vi "Main.vi"() -> ()   [LabVIEW 2013]
uses:
  <vilib>/Utility/miscctls.llb/LVFontTypeDef.ctl
panel:
  out "текущий ист.":u8
  in  "SetCurrent":dbl min=0.0 max=72.0 step=0.1 format="%#.1g"
  in  "SetVoltage":dbl min=0.0 max=30.0 step=0.1 format="%#.1g"
  in  "SetCurrentB":bool
  in  "SetVoltageB":bool
  in  "SetOutputOffB":bool
  in  "SetOutputOnB":bool
  in  "ConnectChannel":bool
  in  "DisconnectChannel":bool
  in  "Comm. current %":dbl=0.5 caption="%" min=0.0 max=100.0 step=0.5
  in  "Common curr. dec":bool
  in  "Common curr. inc":bool
  in  "ConnectAll":bool
  in  "DisconnectAll":bool
  in  "Set Output ON All":bool caption="ВЫХОДЫ ИСТОЧНИКОВ"
  in  "SetCurrentAll":bool
  in  "SetVoltageAll":bool
  out "Дата":string
  out "Время":string
  in  "Comm. voltage %":dbl caption="%" min=0.0 max=100.0 step=0.5
  in  "Common volt. dec":bool
  in  "Common volt. inc":bool
  in  "ReadFromFile":bool
  in  "WriteToFile":bool
  in  "№":string="55"
  in  "DeleteChannel":bool
  in  "IP":string="172.16.21.19"
  in  "AddChannel":bool
  out "CURRENTSET":dbl[](array[numeric])
  in  "CurrentModulationOn":bool
  in  "Amp":dbl
  in  "CurrentModulationB":bool
  out "NAME":string[](array[string])
  out "ADRESS":string[](array[string])
  out "VIRef":refnum<vi>[](array[refnum])
  in  "Quit":bool
  in  "List of channels":i32(listbox)
  # "ИСТОЧНИК №_"
  # "ВСЕ ИСТОЧНИКИ"
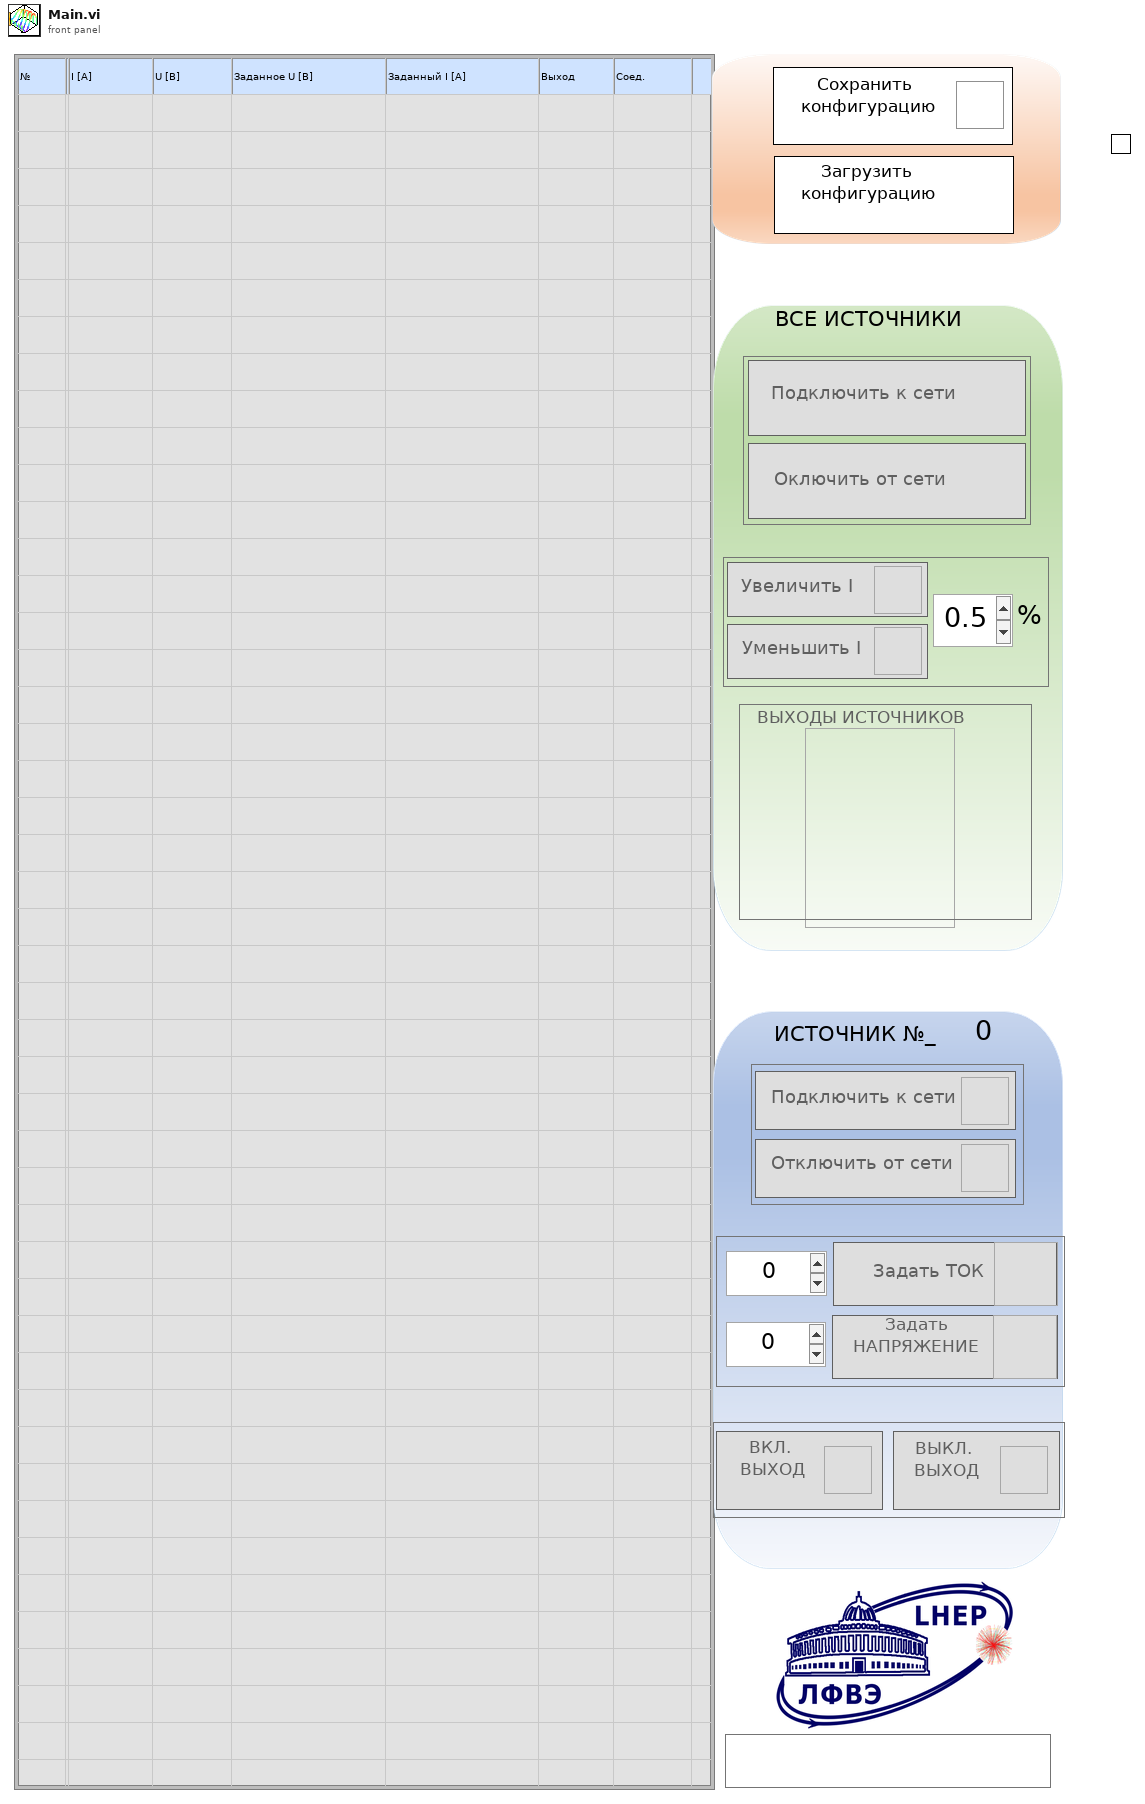
[diagram p1: front panel]
types:
  T1 = enum8{"Enabled", "Disabled", "Disabled and Grayed Out"}
  T2 = typedef "LVFontTypeDef.ctl" = cluster{"Font Name":string, "Size":u16, "Bold":bool, "Italic":bool, "Underline":bool, "Strikeout":bool, "Color":u32}
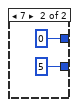
[diagram p4: hidden frame]
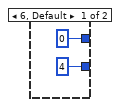
[diagram p5: hidden frame]
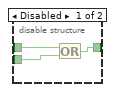
[diagram p6: hidden frame]
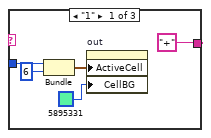
[diagram p7: hidden frame]
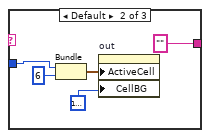
[diagram p8: hidden frame]
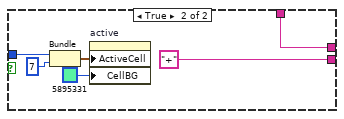
[diagram p9: hidden frame]
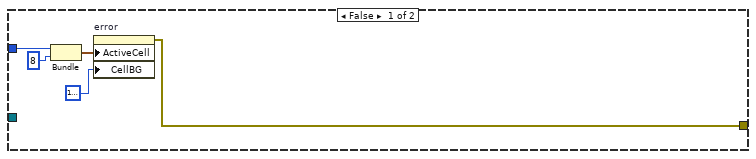
[diagram p10: hidden frame]
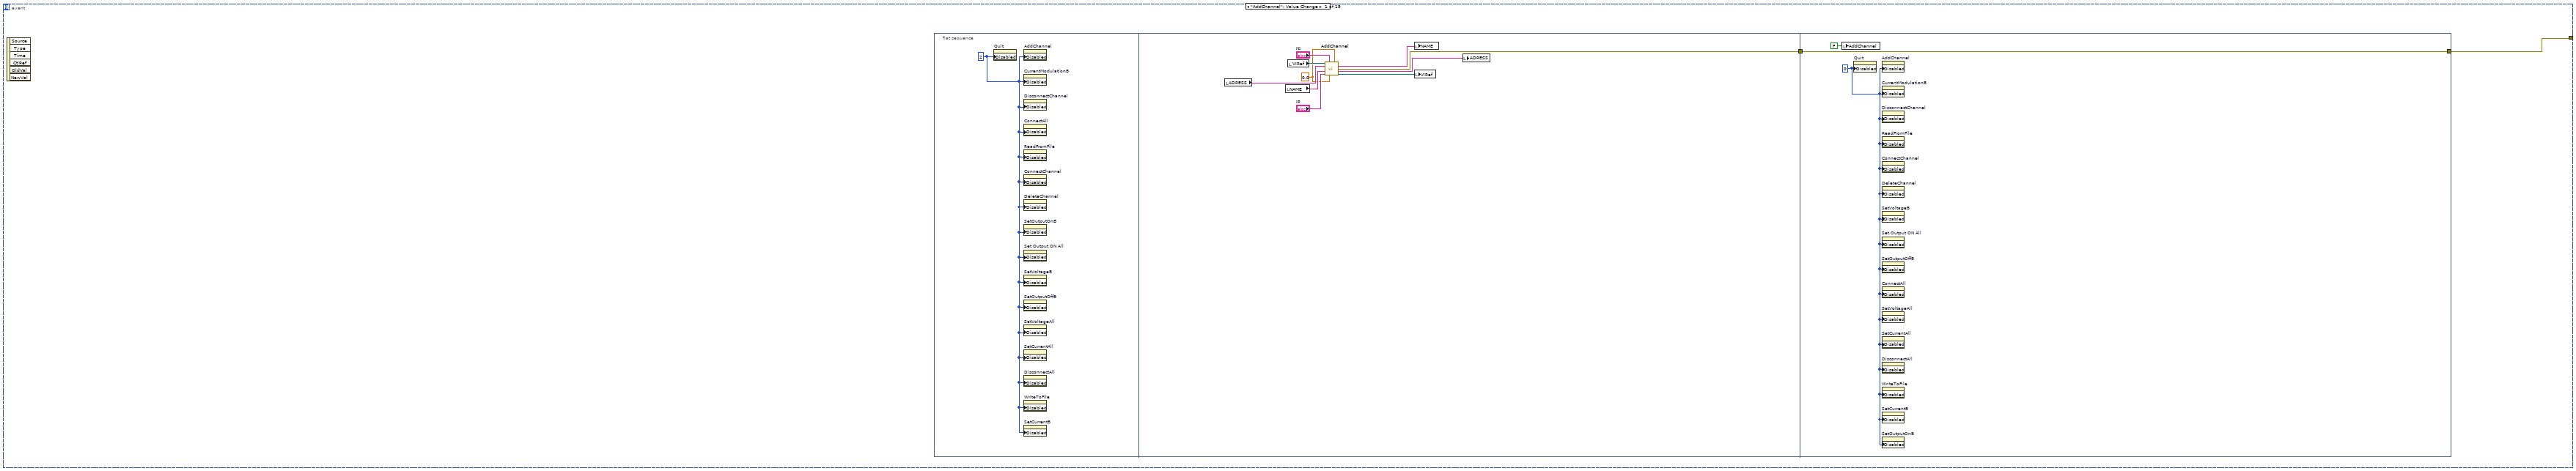
[diagram p11: hidden frame]
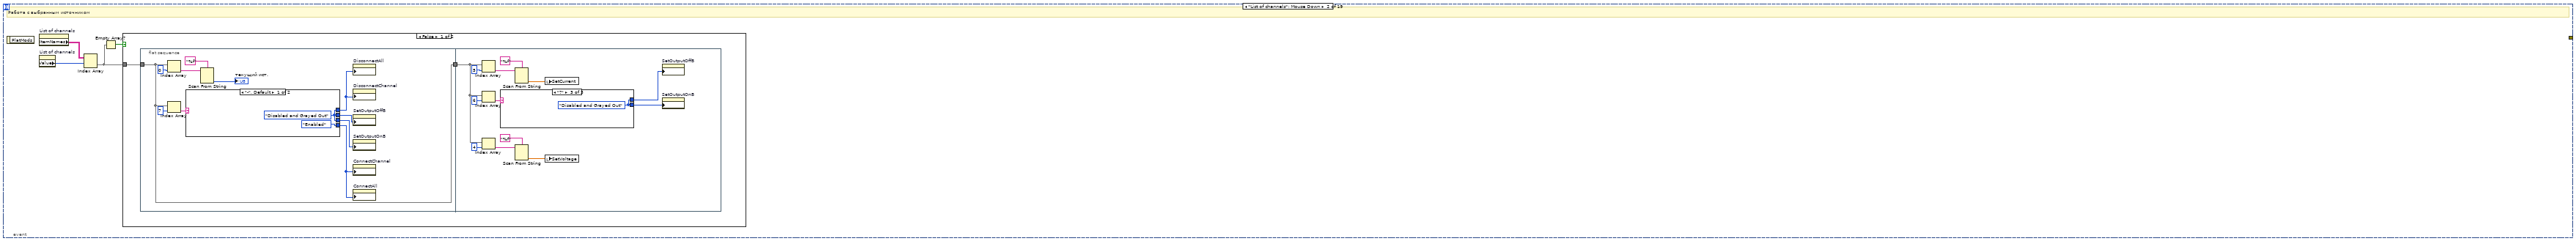
[diagram p12: hidden frame]
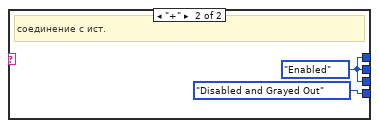
[diagram p13: hidden frame]
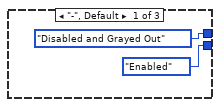
[diagram p14: hidden frame]
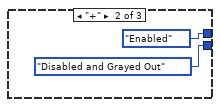
[diagram p15: hidden frame]
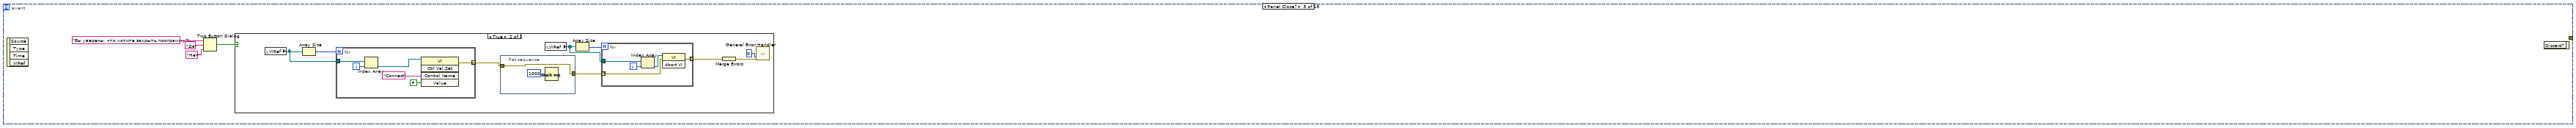
[diagram p17: hidden frame]
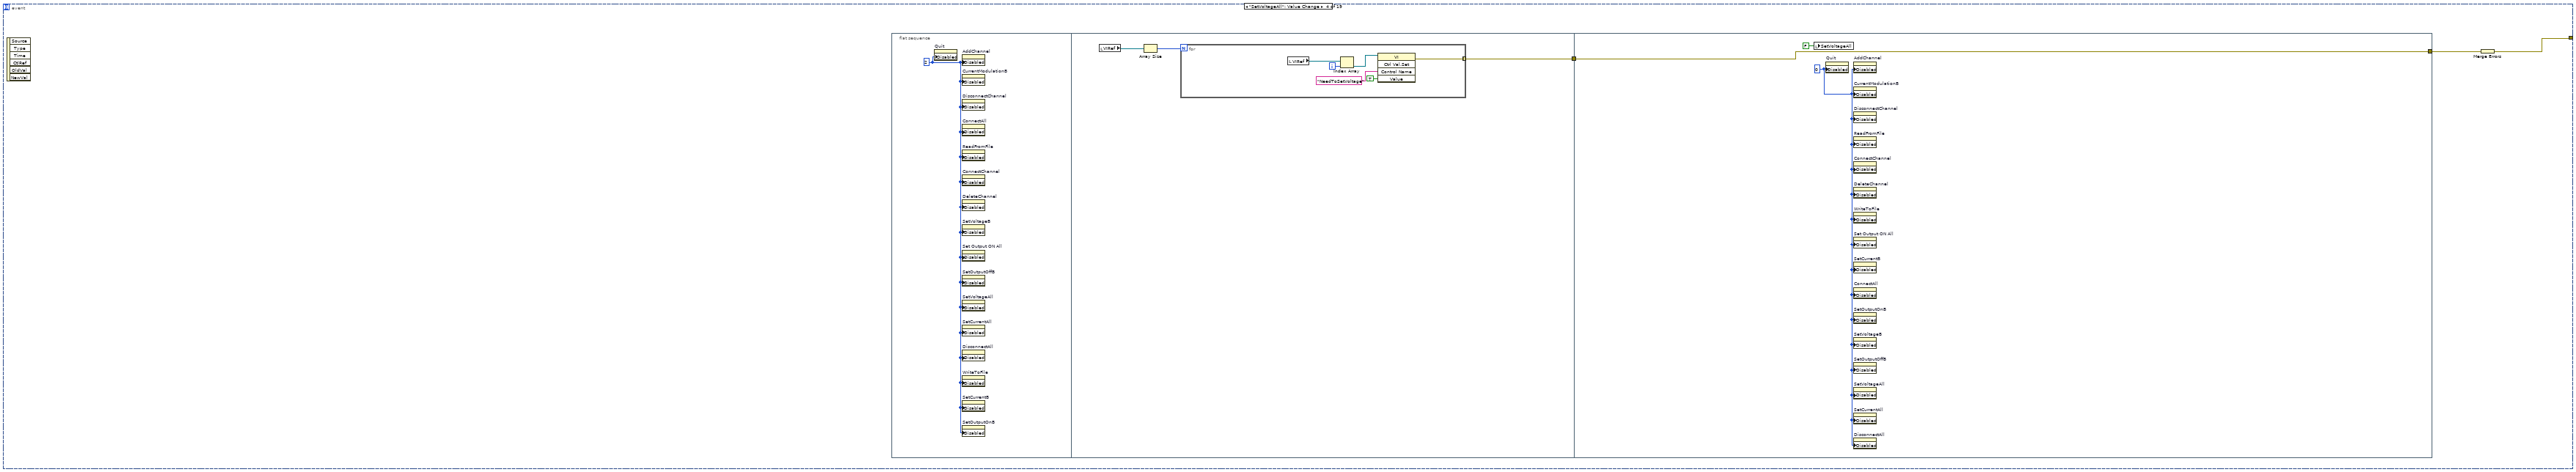
[diagram p19: hidden frame]
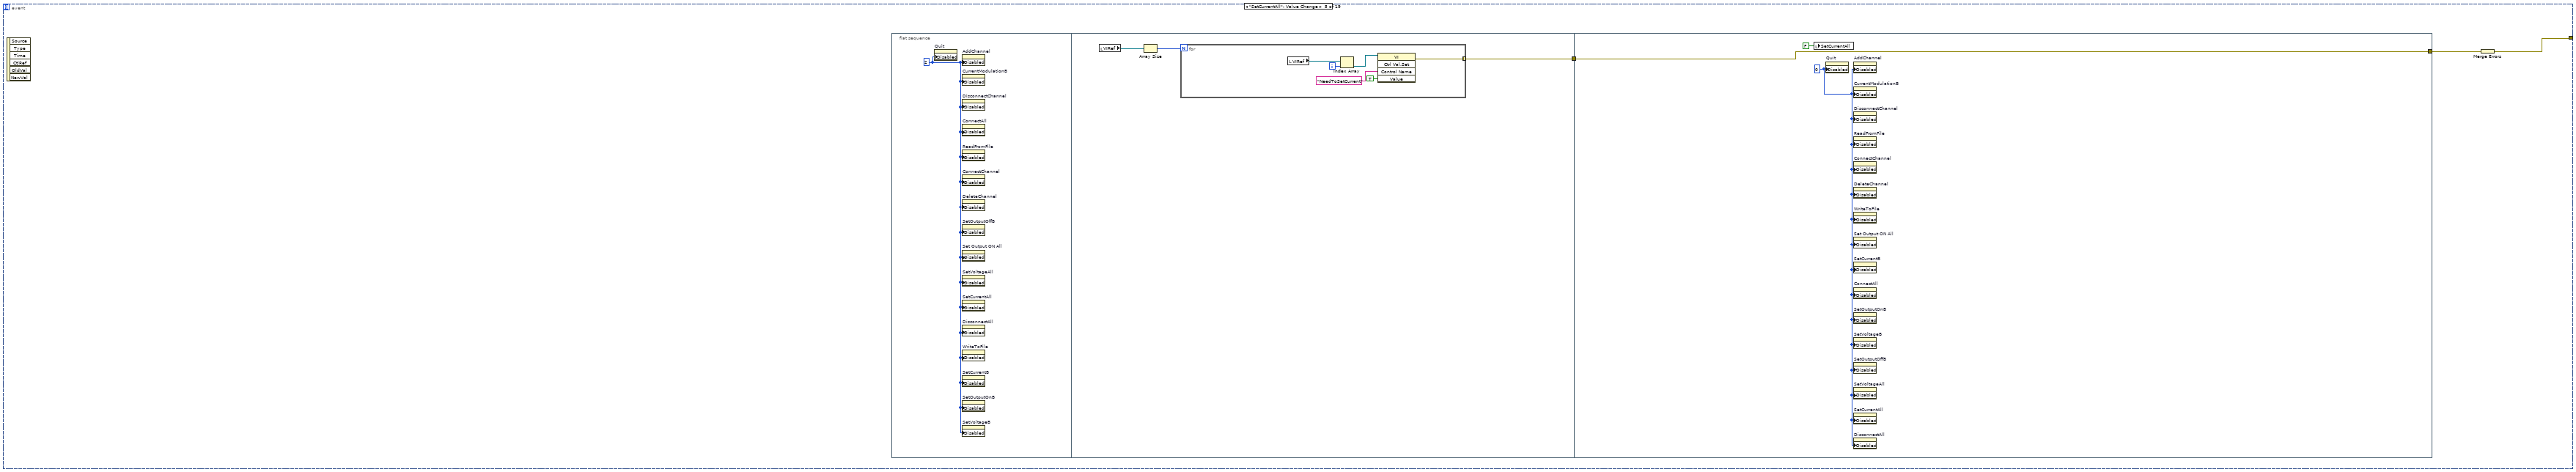
[diagram p20: hidden frame]
diagram:
  w19 = u8 0 ("Disabled")
  w21 = FALSE ("SetOutputOnB")
  w22 = FALSE ("OK Button")
  n1 = event shown="[0] \"Quit\": Value Change" {
    selector: _ -> [_]
    dyn-events: _ -> [_]
    timeout: _ -> [_]
    event "Quit": Value Change {
      n2 = event-data() -> ()  [unwired: 1 in, 5 out]
      n3 = Stop(stop? (T)=TRUE) -> ()
    }
  }
  n4 = while {
    stop <- FALSE stop-if-true
    n5 = property on="List of channels" class="MCListbox (strict)"() -> ("ItemNames"=w33:string[][])  [unwired: 2 in, 2 out]
    n6 = Get Date/Time String(want seconds? (F)=TRUE) -> (date string=→"Дата":string, time string=→"Время":string)  [unwired: 2 in]
    n7 = Wait Until Next ms Multiple(millisecond multiple=u16 1000) -> ()  [unwired: 1 out]
    n8 = Empty Array?(array=w33) -> (empty?=w32:bool)
    n9 = case shown="True" w32 {
      frame False {
      }
      frame True {
        w35 = T1."Disabled and Grayed Out" ("Disabled")
        n10 = property on="Common curr. inc" class="Bool (strict)"("DisabledEnum"=w35) -> ()  [unwired: 2 in, 2 out]
        n11 = property on="Common curr. dec" class="Bool (strict)"("DisabledEnum"=w35) -> ()  [unwired: 2 in, 2 out]
        n12 = property on="Set Output ON All" class="Bool (strict)"("DisabledEnum"=w35) -> ()  [unwired: 2 in, 2 out]
        n13 = property on="Common volt. inc" class="Bool (strict)"("DisabledEnum"=w35) -> ()  [unwired: 2 in, 2 out]
        n14 = property on="DisconnectAll" class="Bool (strict)"("DisabledEnum"=w35) -> ()  [unwired: 2 in, 2 out]
        n15 = property on="SetVoltageB" class="Bool (strict)"("DisabledEnum"=w35) -> ()  [unwired: 2 in, 2 out]
        n16 = property on="ConnectChannel" class="Bool (strict)"("DisabledEnum"=w35) -> ()  [unwired: 2 in, 2 out]
        n17 = property on="SetOutputOnB" class="Bool (strict)"("DisabledEnum"=w35) -> ()  [unwired: 2 in, 2 out]
        n18 = property on="DisconnectChannel" class="Bool (strict)"("DisabledEnum"=w35) -> ()  [unwired: 2 in, 2 out]
        n19 = property on="SetOutputOffB" class="Bool (strict)"("DisabledEnum"=w35) -> ()  [unwired: 2 in, 2 out]
        n20 = property on="ConnectAll" class="Bool (strict)"("DisabledEnum"=w35) -> ()  [unwired: 2 in, 2 out]
        n21 = property on="SetCurrentB" class="Bool (strict)"("DisabledEnum"=w35) -> ()  [unwired: 2 in, 2 out]
      }
    }
  }
  n22 = while {
    stop <- FALSE stop-if-true
    n23 = event shown="[15] \"WriteToFile\": Value Change" {
      selector: _ -> [_ _ _ _ _ _ _ _ _ _ _ _ _ _ _ _ _ _ _]
      dyn-events: _ -> [_ _ _ _ _ _ _ _ _ _ _ _ _ _ _ _ _ _ _]
      timeout: _ -> [_ _ _ _ _ _ _ _ _ _ _ _ _ _ _ _ _ _ _]
      tunnel: [w39 _ _ w120 w136 w152 w196 w240 w255 w281 w297 w313 w330 w351 w374 w392 w443 w517 w540] -> w36
      event "AddChannel": Value Change {
        n24 = event-data() -> ()  [unwired: 7 out]
        n25 = flat-sequence {
          tunnel: [w42] -> w40
          tunnel: [w52] -> w39
          tunnel: w40 -> [w52]
          frame #0 {
            w41 = u8 2 ("Disabled")
            n26 = property on="Quit" class="Bool (strict)"("Disabled"=w41) -> ()  [unwired: 2 in, 2 out]
            n27 = property on="AddChannel" class="Bool (strict)"("Disabled"=w41) -> ()  [unwired: 2 in, 2 out]
            n28 = property on="CurrentModulationB" class="Bool (strict)"("Disabled"=w41) -> ()  [unwired: 2 in, 2 out]
            n29 = property on="DisconnectChannel" class="Bool (strict)"("Disabled"=w41) -> ()  [unwired: 2 in, 2 out]
            n30 = property on="ConnectAll" class="Bool (strict)"("Disabled"=w41) -> ()  [unwired: 2 in, 2 out]
            n31 = property on="ReadFromFile" class="Bool (strict)"("Disabled"=w41) -> ()  [unwired: 2 in, 2 out]
            n32 = property on="ConnectChannel" class="Bool (strict)"("Disabled"=w41) -> ()  [unwired: 2 in, 2 out]
            n33 = property on="DeleteChannel" class="Bool (strict)"("Disabled"=w41) -> ()  [unwired: 2 in, 2 out]
            n34 = property on="SetOutputOnB" class="Bool (strict)"("Disabled"=w41) -> ()  [unwired: 2 in, 2 out]
            n35 = property on="Set Output ON All" class="Bool (strict)"("Disabled"=w41) -> ()  [unwired: 2 in, 2 out]
            n36 = property on="SetVoltageB" class="Bool (strict)"("Disabled"=w41) -> ()  [unwired: 2 in, 2 out]
            n37 = property on="SetOutputOffB" class="Bool (strict)"("Disabled"=w41) -> ()  [unwired: 2 in, 2 out]
            n38 = property on="SetVoltageAll" class="Bool (strict)"("Disabled"=w41) -> ()  [unwired: 2 in, 2 out]
            n39 = property on="SetCurrentAll" class="Bool (strict)"("Disabled"=w41) -> ()  [unwired: 2 in, 2 out]
            n40 = property on="DisconnectAll" class="Bool (strict)"("Disabled"=w41) -> ()  [unwired: 2 in, 2 out]
            n41 = property on="WriteToFile" class="Bool (strict)"("Disabled"=w41) -> ()  [unwired: 2 in, 2 out]
            n42 = property on="SetCurrentB" class="Bool (strict)"("Disabled"=w41) -> ()  [unwired: 2 in, 2 out]
          }
          frame #1 {
            w43 = 0.0 ("SetVoltage")
            n43 = local read "ADRESS"() -> (w49:string[])
            n44 = local read "NAME"() -> (w48:string[])
            n45 = local read "VIRef"() -> (w47:refnum<vi>[])
            n46 = call "AddChannel.vi"("VIRef"=w47, "Name"="№", "SetCurrent"=w43, "ADRESS"=w49, "NAME"=w48, "Address"="IP", "SetVoltage"=w43) -> ("NAMEOut"=w44:string[], "error out"=w42:errorcluster, "ADRESSOut"=w45:string[], "VIRefOut"=w46:refnum<vi>[])  [unwired: 1 in, 4 out]
            n47 = local write "NAME"(w44) -> ()
            n48 = local write "VIRef"(w46) -> ()
            n49 = local write "ADRESS"(w45) -> ()
          }
          frame #2 {
            w53 = u8 0 ("Disabled")
            n50 = local write "AddChannel"(FALSE ("AddChannel")) -> ()
            n51 = property on="Quit" class="Bool (strict)"("Disabled"=w53) -> ()  [unwired: 2 in, 2 out]
            n52 = property on="AddChannel" class="Bool (strict)"("Disabled"=w53) -> ()  [unwired: 2 in, 2 out]
            n53 = property on="CurrentModulationB" class="Bool (strict)"("Disabled"=w53) -> ()  [unwired: 2 in, 2 out]
            n54 = property on="DisconnectChannel" class="Bool (strict)"("Disabled"=w53) -> ()  [unwired: 2 in, 2 out]
            n55 = property on="ReadFromFile" class="Bool (strict)"("Disabled"=w53) -> ()  [unwired: 2 in, 2 out]
            n56 = property on="ConnectChannel" class="Bool (strict)"("Disabled"=w53) -> ()  [unwired: 2 in, 2 out]
            n57 = property on="DeleteChannel" class="Bool (strict)"("Disabled"=w53) -> ()  [unwired: 2 in, 2 out]
            n58 = property on="SetVoltageB" class="Bool (strict)"("Disabled"=w53) -> ()  [unwired: 2 in, 2 out]
            n59 = property on="Set Output ON All" class="Bool (strict)"("Disabled"=w53) -> ()  [unwired: 2 in, 2 out]
            n60 = property on="SetOutputOffB" class="Bool (strict)"("Disabled"=w53) -> ()  [unwired: 2 in, 2 out]
            n61 = property on="ConnectAll" class="Bool (strict)"("Disabled"=w53) -> ()  [unwired: 2 in, 2 out]
            n62 = property on="SetVoltageAll" class="Bool (strict)"("Disabled"=w53) -> ()  [unwired: 2 in, 2 out]
            n63 = property on="SetCurrentAll" class="Bool (strict)"("Disabled"=w53) -> ()  [unwired: 2 in, 2 out]
            n64 = property on="DisconnectAll" class="Bool (strict)"("Disabled"=w53) -> ()  [unwired: 2 in, 2 out]
            n65 = property on="WriteToFile" class="Bool (strict)"("Disabled"=w53) -> ()  [unwired: 2 in, 2 out]
            n66 = property on="SetCurrentB" class="Bool (strict)"("Disabled"=w53) -> ()  [unwired: 2 in, 2 out]
            n67 = property on="SetOutputOnB" class="Bool (strict)"("Disabled"=w53) -> ()  [unwired: 2 in, 2 out]
          }
        }
      }
      event "List of channels": Mouse Down {
        # "Работа с выбранным источником"
        n68 = event-data() -> ()  [unwired: 2 out]
        n69 = property on="List of channels" class="MCListbox (strict)"() -> ("ItemNames"=w58:string[][])  [unwired: 2 in, 2 out]
        n70 = property on="List of channels" class="MCListbox (strict)"() -> ("Value"=w57:i32)  [unwired: 2 in, 2 out]
        n71 = Index Array(array=w58, index (row)=w57) -> (element=w56:string[])  [unwired: 1 in]
        n72 = Empty Array?(array=w56) -> (empty?=w55:bool)
        n73 = case shown="False" w55 {
          tunnel: w56 -> [w59 _]
          frame False {
            n74 = flat-sequence {
              tunnel: w59 -> [w65]
              tunnel: [w65] -> w60
              tunnel: w60 -> [w76]
              frame #0 {
                n75 = Index Array(array=w65, index=0) -> (element=w68:string)
                n76 = Index Array(array=w65, index=7) -> (element=w66:string)
                n77 = case shown="\"-\", Default" w66 {
                  tunnel: [T1."Enabled" ("Disabled") T1."Disabled and Grayed Out" ("Disabled")] -> w61
                  tunnel: [w72 w74] -> w62
                  tunnel: [w72 w74] -> w64
                  tunnel: [w72 w74] -> w63
                  frame "-", Default {
                    w72 = T1."Disabled and Grayed Out" ("Disabled")
                  }
                  frame "+" {
                    w74 = T1."Enabled" ("Disabled")
                    # "соединение с ист."
                  }
                }
                n78 = Scan From String(format string="%f", input string=w68) -> (output 1=→"текущий ист.":u8)  [unwired: 3 in, 3 out]
                n79 = property on="DisconnectAll" class="Bool (strict)"("DisabledEnum"=w62) -> ()  [unwired: 2 in, 2 out]
                n80 = property on="DisconnectChannel" class="Bool (strict)"("DisabledEnum"=w62) -> ()  [unwired: 2 in, 2 out]
                n81 = property on="SetOutputOffB" class="Bool (strict)"("DisabledEnum"=w64) -> ()  [unwired: 2 in, 2 out]
                n82 = property on="SetOutputOnB" class="Bool (strict)"("DisabledEnum"=w63) -> ()  [unwired: 2 in, 2 out]
                n83 = property on="ConnectChannel" class="Bool (strict)"("DisabledEnum"=w61) -> ()  [unwired: 2 in, 2 out]
                n84 = property on="ConnectAll" class="Bool (strict)"("DisabledEnum"=w61) -> ()  [unwired: 2 in, 2 out]
              }
              frame #1 {
                n85 = Index Array(array=w76, index=5) -> (element=w82:string)
                n86 = Index Array(array=w76, index=6) -> (element=w86:string)
                n87 = Index Array(array=w76, index=4) -> (element=w78:string)
                n88 = case shown="\"?\"" w86 {
                  tunnel: [T1."Enabled" ("Disabled") T1."Disabled and Grayed Out" ("Disabled") w93] -> w87
                  tunnel: [T1."Disabled and Grayed Out" ("Disabled") T1."Enabled" ("Disabled") w93] -> w88
                  frame "-", Default {
                  }
                  frame "+" {
                  }
                  frame "?" {
                    w93 = T1."Disabled and Grayed Out" ("Disabled")
                  }
                }
                n89 = Scan From String(format string="%f", input string=w82) -> (output 1=w84:dbl)  [unwired: 3 in, 3 out]
                n90 = Scan From String(format string="%f", input string=w78) -> (output 1=w79:dbl)  [unwired: 3 in, 3 out]
                n91 = local write "SetCurrent"(w84) -> ()
                n92 = local write "SetVoltage"(w79) -> ()
                n93 = property on="SetOutputOffB" class="Bool (strict)"("DisabledEnum"=w88) -> ()  [unwired: 2 in, 2 out]
                n94 = property on="SetOutputOnB" class="Bool (strict)"("DisabledEnum"=w87) -> ()  [unwired: 2 in, 2 out]
              }
            }
          }
          frame True {
          }
        }
      }
      event Panel Close? {
        n95 = event-data() -> ()  [unwired: 5 out]
        n96 = Two Button Dialog(message="Вы уверены, что хотите закрыть программу?", 1:"Нет" ("F button name (\"Cancel\")"), 2:"Да" ("T button name (\"OK\")")) -> (T button?=w97:bool)
        n97 = case shown="True" w97 {
          frame False {
          }
          frame True {
            n98 = local read "VIRef"() -> (w99:refnum<vi>[])
            n99 = Array Size(array=w99) -> (size(s)=w98:i32)
            n100 = for {
              N: w98 -> [_]
              tunnel: w99 -> [w116]
              tunnel: [w114] -> w106 mode=indexing
              i -> [w117]
              n101 = Index Array(array=w116, index=w117) -> (element=w115:refnum<vi>)
              n102 = invoke class="VI" method="Ctrl Val.Set"(reference=w115, "Control Name"="Connect", "Value"=FALSE) -> (error out=w114:errorcluster)  [unwired: 2 in, 4 out]
            }
            n103 = flat-sequence {
              tunnel: [w108] -> w105
              tunnel: w106 -> [w108]
              frame #0 {
                n104 = Wait (ms)(milliseconds to wait=u32 1000) -> ()  [unwired: 1 out]
              }
            }
            n105 = local read "VIRef"() -> (w100:refnum<vi>[])
            n106 = Array Size(array=w100) -> (size(s)=w101:i32)
            n107 = for {
              N: w101 -> [_]
              tunnel: w100 -> [w112]
              tunnel: [w110] -> w102 mode=indexing
              tunnel: w105 -> [w109] mode=indexing
              i -> [w113]
              n108 = Index Array(array=w112, index=w113) -> (element=w111:refnum<vi>)
              n109 = invoke class="VI" method="Abort VI"(reference=w111, error in=w109) -> (error out=w110:errorcluster)  [unwired: 1 in, 2 out]
            }
            n110 = Merge Errors(w102) -> (w103:errorcluster)
            n111 = call <vilib>:"General Error Handler.vi"("type of dialog (OK msg:1)"=u32 0 ("milliseconds to wait"), "error in (no error)"=w103) -> ()  [unwired: 9 in, 5 out]
          }
        }
        n112 = event-data() -> ()  [unwired: 2 in, 1 out]
      }
      event "SetVoltageAll": Value Change {
        n113 = event-data() -> ()  [unwired: 7 out]
        n114 = flat-sequence {
          tunnel: [w124] -> w122
          tunnel: [w133] -> w121
          tunnel: w122 -> [w133]
          frame #0 {
            w123 = u8 2 ("Disabled")
            n115 = property on="Quit" class="Bool (strict)"("Disabled"=w123) -> ()  [unwired: 2 in, 2 out]
            n116 = property on="AddChannel" class="Bool (strict)"("Disabled"=w123) -> ()  [unwired: 2 in, 2 out]
            n117 = property on="CurrentModulationB" class="Bool (strict)"("Disabled"=w123) -> ()  [unwired: 2 in, 2 out]
            n118 = property on="DisconnectChannel" class="Bool (strict)"("Disabled"=w123) -> ()  [unwired: 2 in, 2 out]
            n119 = property on="ConnectAll" class="Bool (strict)"("Disabled"=w123) -> ()  [unwired: 2 in, 2 out]
            n120 = property on="ReadFromFile" class="Bool (strict)"("Disabled"=w123) -> ()  [unwired: 2 in, 2 out]
            n121 = property on="ConnectChannel" class="Bool (strict)"("Disabled"=w123) -> ()  [unwired: 2 in, 2 out]
            n122 = property on="DeleteChannel" class="Bool (strict)"("Disabled"=w123) -> ()  [unwired: 2 in, 2 out]
            n123 = property on="SetVoltageB" class="Bool (strict)"("Disabled"=w123) -> ()  [unwired: 2 in, 2 out]
            n124 = property on="Set Output ON All" class="Bool (strict)"("Disabled"=w123) -> ()  [unwired: 2 in, 2 out]
            n125 = property on="SetOutputOffB" class="Bool (strict)"("Disabled"=w123) -> ()  [unwired: 2 in, 2 out]
            n126 = property on="SetVoltageAll" class="Bool (strict)"("Disabled"=w123) -> ()  [unwired: 2 in, 2 out]
            n127 = property on="SetCurrentAll" class="Bool (strict)"("Disabled"=w123) -> ()  [unwired: 2 in, 2 out]
            n128 = property on="DisconnectAll" class="Bool (strict)"("Disabled"=w123) -> ()  [unwired: 2 in, 2 out]
            n129 = property on="WriteToFile" class="Bool (strict)"("Disabled"=w123) -> ()  [unwired: 2 in, 2 out]
            n130 = property on="SetCurrentB" class="Bool (strict)"("Disabled"=w123) -> ()  [unwired: 2 in, 2 out]
            n131 = property on="SetOutputOnB" class="Bool (strict)"("Disabled"=w123) -> ()  [unwired: 2 in, 2 out]
          }
          frame #1 {
            n132 = local read "VIRef"() -> (w126:refnum<vi>[])
            n133 = Array Size(array=w126) -> (size(s)=w125:i32)
            n134 = for {
              N: w125 -> [_]
              tunnel: [w127] -> w124 mode=indexing
              i -> [w129]
              n135 = local read "VIRef"() -> (w132:refnum<vi>[])
              n136 = Index Array(array=w132, index=w129) -> (element=w128:refnum<vi>)
              n137 = invoke class="VI" method="Ctrl Val.Set"(reference=w128, "Control Name"="NeedToSetVoltage", "Value"=TRUE ("ConnectChannel")) -> (error out=w127:errorcluster)  [unwired: 2 in, 4 out]
            }
          }
          frame #2 {
            w134 = u8 0 ("Disabled")
            n138 = local write "SetVoltageAll"(FALSE ("SetVoltageAll")) -> ()
            n139 = property on="Quit" class="Bool (strict)"("Disabled"=w134) -> ()  [unwired: 2 in, 2 out]
            n140 = property on="AddChannel" class="Bool (strict)"("Disabled"=w134) -> ()  [unwired: 2 in, 2 out]
            n141 = property on="CurrentModulationB" class="Bool (strict)"("Disabled"=w134) -> ()  [unwired: 2 in, 2 out]
            n142 = property on="DisconnectChannel" class="Bool (strict)"("Disabled"=w134) -> ()  [unwired: 2 in, 2 out]
            n143 = property on="ReadFromFile" class="Bool (strict)"("Disabled"=w134) -> ()  [unwired: 2 in, 2 out]
            n144 = property on="ConnectChannel" class="Bool (strict)"("Disabled"=w134) -> ()  [unwired: 2 in, 2 out]
            n145 = property on="DeleteChannel" class="Bool (strict)"("Disabled"=w134) -> ()  [unwired: 2 in, 2 out]
            n146 = property on="WriteToFile" class="Bool (strict)"("Disabled"=w134) -> ()  [unwired: 2 in, 2 out]
            n147 = property on="Set Output ON All" class="Bool (strict)"("Disabled"=w134) -> ()  [unwired: 2 in, 2 out]
            n148 = property on="SetCurrentB" class="Bool (strict)"("Disabled"=w134) -> ()  [unwired: 2 in, 2 out]
            n149 = property on="ConnectAll" class="Bool (strict)"("Disabled"=w134) -> ()  [unwired: 2 in, 2 out]
            n150 = property on="SetOutputOnB" class="Bool (strict)"("Disabled"=w134) -> ()  [unwired: 2 in, 2 out]
            n151 = property on="SetVoltageB" class="Bool (strict)"("Disabled"=w134) -> ()  [unwired: 2 in, 2 out]
            n152 = property on="SetOutputOffB" class="Bool (strict)"("Disabled"=w134) -> ()  [unwired: 2 in, 2 out]
            n153 = property on="SetVoltageAll" class="Bool (strict)"("Disabled"=w134) -> ()  [unwired: 2 in, 2 out]
            n154 = property on="SetCurrentAll" class="Bool (strict)"("Disabled"=w134) -> ()  [unwired: 2 in, 2 out]
            n155 = property on="DisconnectAll" class="Bool (strict)"("Disabled"=w134) -> ()  [unwired: 2 in, 2 out]
          }
        }
        n156 = Merge Errors(w121) -> (w120:errorcluster)
      }
      event "SetCurrentAll": Value Change {
        n157 = event-data() -> ()  [unwired: 7 out]
        n158 = flat-sequence {
          tunnel: [w140] -> w138
          tunnel: [w149] -> w137
          tunnel: w138 -> [w149]
          frame #0 {
            w139 = u8 2 ("Disabled")
            n159 = property on="Quit" class="Bool (strict)"("Disabled"=w139) -> ()  [unwired: 2 in, 2 out]
            n160 = property on="AddChannel" class="Bool (strict)"("Disabled"=w139) -> ()  [unwired: 2 in, 2 out]
            n161 = property on="CurrentModulationB" class="Bool (strict)"("Disabled"=w139) -> ()  [unwired: 2 in, 2 out]
            n162 = property on="DisconnectChannel" class="Bool (strict)"("Disabled"=w139) -> ()  [unwired: 2 in, 2 out]
            n163 = property on="ConnectAll" class="Bool (strict)"("Disabled"=w139) -> ()  [unwired: 2 in, 2 out]
            n164 = property on="ReadFromFile" class="Bool (strict)"("Disabled"=w139) -> ()  [unwired: 2 in, 2 out]
            n165 = property on="ConnectChannel" class="Bool (strict)"("Disabled"=w139) -> ()  [unwired: 2 in, 2 out]
            n166 = property on="DeleteChannel" class="Bool (strict)"("Disabled"=w139) -> ()  [unwired: 2 in, 2 out]
            n167 = property on="SetOutputOffB" class="Bool (strict)"("Disabled"=w139) -> ()  [unwired: 2 in, 2 out]
            n168 = property on="Set Output ON All" class="Bool (strict)"("Disabled"=w139) -> ()  [unwired: 2 in, 2 out]
            n169 = property on="SetVoltageAll" class="Bool (strict)"("Disabled"=w139) -> ()  [unwired: 2 in, 2 out]
            n170 = property on="SetCurrentAll" class="Bool (strict)"("Disabled"=w139) -> ()  [unwired: 2 in, 2 out]
            n171 = property on="DisconnectAll" class="Bool (strict)"("Disabled"=w139) -> ()  [unwired: 2 in, 2 out]
            n172 = property on="WriteToFile" class="Bool (strict)"("Disabled"=w139) -> ()  [unwired: 2 in, 2 out]
            n173 = property on="SetCurrentB" class="Bool (strict)"("Disabled"=w139) -> ()  [unwired: 2 in, 2 out]
            n174 = property on="SetOutputOnB" class="Bool (strict)"("Disabled"=w139) -> ()  [unwired: 2 in, 2 out]
            n175 = property on="SetVoltageB" class="Bool (strict)"("Disabled"=w139) -> ()  [unwired: 2 in, 2 out]
          }
          frame #1 {
            n176 = local read "VIRef"() -> (w142:refnum<vi>[])
            n177 = Array Size(array=w142) -> (size(s)=w141:i32)
            n178 = for {
              N: w141 -> [_]
              tunnel: [w143] -> w140 mode=indexing
              i -> [w145]
              n179 = local read "VIRef"() -> (w148:refnum<vi>[])
              n180 = Index Array(array=w148, index=w145) -> (element=w144:refnum<vi>)
              n181 = invoke class="VI" method="Ctrl Val.Set"(reference=w144, "Control Name"="NeedToSetCurrent", "Value"=TRUE ("ConnectChannel")) -> (error out=w143:errorcluster)  [unwired: 2 in, 4 out]
            }
          }
          frame #2 {
            w150 = u8 0 ("Disabled")
            n182 = local write "SetCurrentAll"(FALSE ("SetVoltageAll")) -> ()
            n183 = property on="Quit" class="Bool (strict)"("Disabled"=w150) -> ()  [unwired: 2 in, 2 out]
            n184 = property on="AddChannel" class="Bool (strict)"("Disabled"=w150) -> ()  [unwired: 2 in, 2 out]
            n185 = property on="CurrentModulationB" class="Bool (strict)"("Disabled"=w150) -> ()  [unwired: 2 in, 2 out]
            n186 = property on="DisconnectChannel" class="Bool (strict)"("Disabled"=w150) -> ()  [unwired: 2 in, 2 out]
            n187 = property on="ReadFromFile" class="Bool (strict)"("Disabled"=w150) -> ()  [unwired: 2 in, 2 out]
            n188 = property on="ConnectChannel" class="Bool (strict)"("Disabled"=w150) -> ()  [unwired: 2 in, 2 out]
            n189 = property on="DeleteChannel" class="Bool (strict)"("Disabled"=w150) -> ()  [unwired: 2 in, 2 out]
            n190 = property on="WriteToFile" class="Bool (strict)"("Disabled"=w150) -> ()  [unwired: 2 in, 2 out]
            n191 = property on="Set Output ON All" class="Bool (strict)"("Disabled"=w150) -> ()  [unwired: 2 in, 2 out]
            n192 = property on="SetCurrentB" class="Bool (strict)"("Disabled"=w150) -> ()  [unwired: 2 in, 2 out]
            n193 = property on="ConnectAll" class="Bool (strict)"("Disabled"=w150) -> ()  [unwired: 2 in, 2 out]
            n194 = property on="SetOutputOnB" class="Bool (strict)"("Disabled"=w150) -> ()  [unwired: 2 in, 2 out]
            n195 = property on="SetVoltageB" class="Bool (strict)"("Disabled"=w150) -> ()  [unwired: 2 in, 2 out]
            n196 = property on="SetOutputOffB" class="Bool (strict)"("Disabled"=w150) -> ()  [unwired: 2 in, 2 out]
            n197 = property on="SetVoltageAll" class="Bool (strict)"("Disabled"=w150) -> ()  [unwired: 2 in, 2 out]
            n198 = property on="SetCurrentAll" class="Bool (strict)"("Disabled"=w150) -> ()  [unwired: 2 in, 2 out]
            n199 = property on="DisconnectAll" class="Bool (strict)"("Disabled"=w150) -> ()  [unwired: 2 in, 2 out]
          }
        }
        n200 = Merge Errors(w137) -> (w136:errorcluster)
      }
      event "Common curr. inc", "Common curr. dec": Value Change {
        # "Общее управление токами"
        n201 = event-data() -> ()  [unwired: 2 out]
        n202 = local read "ADRESS"() -> (w155:string[])
        n203 = Array Size(array=w155) -> (size(s)=w156:i32)
        n204 = for {
          N: w156 -> [_]
          tunnel: [w165] -> w154 mode=indexing
          i -> [w183]
          n205 = local read "VIRef"() -> (w186:refnum<vi>[])
          n206 = Index Array(array=w186, index=w183) -> (element=w173:refnum<vi>)
          n207 = invoke class="VI" method="Ctrl Val.Get"(reference=w173, "Control Name"="SetCurrentStr") -> (reference out=w167:refnum<vi>, error out=w181:errorcluster, "Get Control Value Variant"=w185:variant)  [unwired: 2 in, 1 out]
          n208 = Variant To Data(error in=w181, type="" ("Control Name"), Variant=w185) -> (data=w180:string, error out=w179:errorcluster)
          n209 = Scan From String(format string="%f", input string=w180, error in=w179) -> (error out=w166:errorcluster, output 1=w164:dbl)  [unwired: 2 in, 2 out]
          n210 = Multiply(x=w164, y="Comm. current %") -> (x*y=w175:dbl)
          n211 = Divide(x=w175, y=100.0) -> (x/y=w177:dbl)
          n212 = local read "Common curr. inc"() -> (w163:bool)
          n213 = local read "Common curr. dec"() -> (w161:bool)
          n214 = case shown="True" w163 {
            tunnel: w177 -> [w191 w195]
            tunnel: w164 -> [w192 w194]
            tunnel: [w192 w193] -> w162
            tunnel: [w191 _] -> w160
            frame False {
            }
            frame True {
              n215 = Add(x=w194, y=w195) -> (x+y=w193:dbl)
            }
          }
          n216 = case shown="False" w161 {
            tunnel: w162 -> [w187 w190]
            tunnel: [w187 w189] -> w159
            tunnel: w160 -> [_ w188]
            frame False {
            }
            frame True {
              n217 = Subtract(x=w190, y=w188) -> (x-y=w189:dbl)
            }
          }
          n218 = invoke class="VI" method="Ctrl Val.Set"(reference=w167, error in=w166, "Control Name"="SetCurrent", "Value"=w159) -> (reference out=w169:refnum<vi>, error out=w168:errorcluster)  [unwired: 1 in, 3 out]
          n219 = invoke class="VI" method="Ctrl Val.Set"(reference=w169, error in=w168, "Control Name"="NeedToSetCurrent", "Value"=TRUE ("ConnectChannel")) -> (error out=w165:errorcluster)  [unwired: 1 in, 4 out]
        }
        n220 = Merge Errors(w154) -> (w153:errorcluster)
        n221 = flat-sequence {
          tunnel: w153 -> [w158]
          tunnel: [w158] -> w152
          frame #0 {
            w157 = FALSE ("ConnectChannel")
            n222 = local write "Common curr. inc"(w157) -> ()
            n223 = local write "Common curr. dec"(w157) -> ()
          }
        }
      }
      event "Common volt. inc", "Common volt. dec": Value Change {
        # "Общее управление напряжением"
        n224 = event-data() -> ()  [unwired: 2 out]
        n225 = local read "ADRESS"() -> (w199:string[])
        n226 = Array Size(array=w199) -> (size(s)=w200:i32)
        n227 = for {
          N: w200 -> [_]
          tunnel: [w210] -> w198 mode=indexing
          i -> [w227]
          n228 = local read "VIRef"() -> (w230:refnum<vi>[])
          n229 = Index Array(array=w230, index=w227) -> (element=w218:refnum<vi>)
          n230 = invoke class="VI" method="Ctrl Val.Get"(reference=w218, "Control Name"="SetVoltageStr") -> (reference out=w212:refnum<vi>, error out=w225:errorcluster, "Get Control Value Variant"=w229:variant)  [unwired: 2 in, 1 out]
          n231 = Variant To Data(error in=w225, type="" ("Control Name"), Variant=w229) -> (data=w224:string, error out=w223:errorcluster)
          n232 = Scan From String(format string="%f", input string=w224, error in=w223) -> (error out=w211:errorcluster, output 1=w209:dbl)  [unwired: 2 in, 2 out]
          n233 = Multiply(x=w209, y="Comm. voltage %") -> (x*y=w219:dbl)
          n234 = Divide(x=w219, y=100.0) -> (x/y=w221:dbl)
          n235 = local read "Common volt. inc"() -> (w208:bool)
          n236 = local read "Common volt. dec"() -> (w206:bool)
          n237 = case shown="True" w208 {
            tunnel: w221 -> [w235 w239]
            tunnel: w209 -> [w236 w238]
            tunnel: [w236 w237] -> w207
            tunnel: [w235 _] -> w205
            frame False {
            }
            frame True {
              n238 = Add(x=w238, y=w239) -> (x+y=w237:dbl)
            }
          }
          n239 = case shown="False" w206 {
            tunnel: w207 -> [w231 w234]
            tunnel: [w231 w233] -> w204
            tunnel: w205 -> [_ w232]
            frame False {
            }
            frame True {
              n240 = Subtract(x=w234, y=w232) -> (x-y=w233:dbl)
            }
          }
          n241 = invoke class="VI" method="Ctrl Val.Set"(reference=w212, error in=w211, "Control Name"="SetVoltage", "Value"=w204) -> (reference out=w214:refnum<vi>, error out=w213:errorcluster)  [unwired: 1 in, 3 out]
          n242 = invoke class="VI" method="Ctrl Val.Set"(reference=w214, error in=w213, "Control Name"="NeedToSetVoltage", "Value"=TRUE ("ConnectChannel")) -> (error out=w210:errorcluster)  [unwired: 1 in, 4 out]
        }
        n243 = Merge Errors(w198) -> (w197:errorcluster)
        n244 = flat-sequence {
          tunnel: w197 -> [w202]
          tunnel: [w202] -> w196
          frame #0 {
            w201 = FALSE ("ConnectChannel")
            n245 = local write "Common volt. inc"(w201) -> ()
            n246 = local write "Common volt. dec"(w201) -> ()
          }
        }
      }
      event "DisconnectChannel": Value Change {
        n247 = event-data() -> ()  [unwired: 7 out]
        n248 = property on="List of channels" class="MCListbox (strict)"() -> ("Value"=w244:i32)  [unwired: 2 in, 2 out]
        n249 = flat-sequence {
          tunnel: w244 -> [w246]
          tunnel: [w246] -> w243
          tunnel: w243 -> [w248]
          tunnel: [w247] -> w241
          tunnel: [w253] -> w242
          tunnel: w241 -> [w253]
          frame #0 {
            w245 = u8 2 ("Disabled")
            n250 = property on="AddChannel" class="Bool (strict)"("Disabled"=w245) -> ()  [unwired: 2 in, 2 out]
            n251 = property on="Set Output ON All" class="Bool (strict)"("Disabled"=w245) -> ()  [unwired: 2 in, 2 out]
            n252 = property on="CurrentModulationB" class="Bool (strict)"("Disabled"=w245) -> ()  [unwired: 2 in, 2 out]
            n253 = property on="ConnectAll" class="Bool (strict)"("Disabled"=w245) -> ()  [unwired: 2 in, 2 out]
            n254 = property on="DisconnectChannel" class="Bool (strict)"("Disabled"=w245) -> ()  [unwired: 2 in, 2 out]
            n255 = property on="ReadFromFile" class="Bool (strict)"("Disabled"=w245) -> ()  [unwired: 2 in, 2 out]
            n256 = property on="Quit" class="Bool (strict)"("Disabled"=w245) -> ()  [unwired: 2 in, 2 out]
            n257 = property on="ConnectChannel" class="Bool (strict)"("Disabled"=w245) -> ()  [unwired: 2 in, 2 out]
            n258 = property on="DeleteChannel" class="Bool (strict)"("Disabled"=w245) -> ()  [unwired: 2 in, 2 out]
            n259 = property on="WriteToFile" class="Bool (strict)"("Disabled"=w245) -> ()  [unwired: 2 in, 2 out]
            n260 = property on="SetCurrentB" class="Bool (strict)"("Disabled"=w245) -> ()  [unwired: 2 in, 2 out]
            n261 = property on="SetOutputOnB" class="Bool (strict)"("Disabled"=w245) -> ()  [unwired: 2 in, 2 out]
            n262 = property on="SetVoltageB" class="Bool (strict)"("Disabled"=w245) -> ()  [unwired: 2 in, 2 out]
            n263 = property on="SetOutputOffB" class="Bool (strict)"("Disabled"=w245) -> ()  [unwired: 2 in, 2 out]
            n264 = property on="SetVoltageAll" class="Bool (strict)"("Disabled"=w245) -> ()  [unwired: 2 in, 2 out]
            n265 = property on="SetCurrentAll" class="Bool (strict)"("Disabled"=w245) -> ()  [unwired: 2 in, 2 out]
            n266 = property on="DisconnectAll" class="Bool (strict)"("Disabled"=w245) -> ()  [unwired: 2 in, 2 out]
          }
          frame #1 {
            w249 = FALSE ("OK Button")
            n267 = local write "DisconnectChannel"(w249) -> ()
            n268 = local read "VIRef"() -> (w251:refnum<vi>[])
            n269 = Index Array(array=w251, index=w248) -> (element=w250:refnum<vi>)
            n270 = invoke class="VI" method="Ctrl Val.Set"(reference=w250, "Control Name"="Connect", "Value"=w249) -> (error out=w247:errorcluster)  [unwired: 2 in, 4 out]
          }
          frame #2 {
            w254 = u8 0 ("Disabled")
            n271 = property on="AddChannel" class="Bool (strict)"("Disabled"=w254) -> ()  [unwired: 2 in, 2 out]
            n272 = property on="CurrentModulationB" class="Bool (strict)"("Disabled"=w254) -> ()  [unwired: 2 in, 2 out]
            n273 = property on="DisconnectChannel" class="Bool (strict)"("Disabled"=w254) -> ()  [unwired: 2 in, 2 out]
            n274 = property on="ConnectAll" class="Bool (strict)"("Disabled"=w254) -> ()  [unwired: 2 in, 2 out]
            n275 = property on="ReadFromFile" class="Bool (strict)"("Disabled"=w254) -> ()  [unwired: 2 in, 2 out]
            n276 = property on="ConnectChannel" class="Bool (strict)"("Disabled"=w254) -> ()  [unwired: 2 in, 2 out]
            n277 = property on="Quit" class="Bool (strict)"("Disabled"=w254) -> ()  [unwired: 2 in, 2 out]
            n278 = property on="DeleteChannel" class="Bool (strict)"("Disabled"=w254) -> ()  [unwired: 2 in, 2 out]
            n279 = property on="SetOutputOffB" class="Bool (strict)"("Disabled"=w254) -> ()  [unwired: 2 in, 2 out]
            n280 = property on="Set Output ON All" class="Bool (strict)"("Disabled"=w254) -> ()  [unwired: 2 in, 2 out]
            n281 = property on="SetVoltageAll" class="Bool (strict)"("Disabled"=w254) -> ()  [unwired: 2 in, 2 out]
            n282 = property on="SetCurrentAll" class="Bool (strict)"("Disabled"=w254) -> ()  [unwired: 2 in, 2 out]
            n283 = property on="DisconnectAll" class="Bool (strict)"("Disabled"=w254) -> ()  [unwired: 2 in, 2 out]
            n284 = property on="WriteToFile" class="Bool (strict)"("Disabled"=w254) -> ()  [unwired: 2 in, 2 out]
            n285 = property on="SetCurrentB" class="Bool (strict)"("Disabled"=w254) -> ()  [unwired: 2 in, 2 out]
            n286 = property on="SetOutputOnB" class="Bool (strict)"("Disabled"=w254) -> ()  [unwired: 2 in, 2 out]
            n287 = property on="SetVoltageB" class="Bool (strict)"("Disabled"=w254) -> ()  [unwired: 2 in, 2 out]
          }
        }
        n288 = Merge Errors(w242) -> (w240:errorcluster)
      }
      event "ConnectChannel": Value Change {
        n289 = event-data() -> ()  [unwired: 7 out]
        n290 = property on="List of channels" class="MCListbox (strict)"() -> ("Value"=w259:i32)  [unwired: 2 in, 2 out]
        n291 = flat-sequence {
          tunnel: w259 -> [w261]
          tunnel: [w261] -> w258
          tunnel: w258 -> [w266]
          tunnel: [w265] -> w256
          tunnel: [w278] -> w257
          tunnel: w256 -> [w278]
          frame #0 {
            w260 = u8 2 ("Disabled")
            n292 = property on="AddChannel" class="Bool (strict)"("Disabled"=w260) -> ()  [unwired: 2 in, 2 out]
            n293 = property on="Set Output ON All" class="Bool (strict)"("Disabled"=w260) -> ()  [unwired: 2 in, 2 out]
            n294 = property on="CurrentModulationB" class="Bool (strict)"("Disabled"=w260) -> ()  [unwired: 2 in, 2 out]
            n295 = property on="ConnectAll" class="Bool (strict)"("Disabled"=w260) -> ()  [unwired: 2 in, 2 out]
            n296 = property on="DisconnectChannel" class="Bool (strict)"("Disabled"=w260) -> ()  [unwired: 2 in, 2 out]
            n297 = property on="ReadFromFile" class="Bool (strict)"("Disabled"=w260) -> ()  [unwired: 2 in, 2 out]
            n298 = property on="Quit" class="Bool (strict)"("Disabled"=w260) -> ()  [unwired: 2 in, 2 out]
            n299 = property on="ConnectChannel" class="Bool (strict)"("Disabled"=w260) -> ()  [unwired: 2 in, 2 out]
            n300 = property on="DeleteChannel" class="Bool (strict)"("Disabled"=w260) -> ()  [unwired: 2 in, 2 out]
            n301 = property on="WriteToFile" class="Bool (strict)"("Disabled"=w260) -> ()  [unwired: 2 in, 2 out]
            n302 = property on="SetCurrentB" class="Bool (strict)"("Disabled"=w260) -> ()  [unwired: 2 in, 2 out]
            n303 = property on="SetOutputOnB" class="Bool (strict)"("Disabled"=w260) -> ()  [unwired: 2 in, 2 out]
            n304 = property on="SetVoltageB" class="Bool (strict)"("Disabled"=w260) -> ()  [unwired: 2 in, 2 out]
            n305 = property on="SetOutputOffB" class="Bool (strict)"("Disabled"=w260) -> ()  [unwired: 2 in, 2 out]
            n306 = property on="SetVoltageAll" class="Bool (strict)"("Disabled"=w260) -> ()  [unwired: 2 in, 2 out]
            n307 = property on="SetCurrentAll" class="Bool (strict)"("Disabled"=w260) -> ()  [unwired: 2 in, 2 out]
            n308 = property on="DisconnectAll" class="Bool (strict)"("Disabled"=w260) -> ()  [unwired: 2 in, 2 out]
          }
          frame #1 {
            n309 = local read "VIRef"() -> (w267:refnum<vi>[])
            n310 = Index Array(array=w267, index=w266) -> (element=w264:refnum<vi>)
            n311 = flat-sequence {
              tunnel: w264 -> [w269]
              tunnel: [w268] -> w262
              tunnel: [w272] -> w263
              tunnel: w262 -> [w272]
              tunnel: [w274] -> w265
              tunnel: w263 -> [w275]
              frame #0 {
                n312 = invoke class="VI" method="Ctrl Val.Set"(reference=w269, "Control Name"="Connect", "Value"=FALSE ("OK Button")) -> (reference out=w268:refnum<vi>)  [unwired: 2 in, 4 out]
              }
              frame #1 {
                n313 = Wait (ms)(milliseconds to wait=u32 1000) -> ()  [unwired: 1 out]
              }
              frame #2 {
                n314 = invoke class="VI" method="Ctrl Val.Set"(reference=w275, "Control Name"="Connect", "Value"=TRUE ("OK Button")) -> (error out=w274:errorcluster)  [unwired: 2 in, 4 out]
              }
            }
          }
          frame #2 {
            w279 = u8 0 ("Disabled")
            n315 = local write "ConnectChannel"(FALSE ("ConnectChannel")) -> ()
            n316 = property on="ConnectAll" class="Bool (strict)"("Disabled"=w279) -> ()  [unwired: 2 in, 2 out]
            n317 = property on="Set Output ON All" class="Bool (strict)"("Disabled"=w279) -> ()  [unwired: 2 in, 2 out]
            n318 = property on="AddChannel" class="Bool (strict)"("Disabled"=w279) -> ()  [unwired: 2 in, 2 out]
            n319 = property on="DisconnectChannel" class="Bool (strict)"("Disabled"=w279) -> ()  [unwired: 2 in, 2 out]
            n320 = property on="ReadFromFile" class="Bool (strict)"("Disabled"=w279) -> ()  [unwired: 2 in, 2 out]
            n321 = property on="ConnectChannel" class="Bool (strict)"("Disabled"=w279) -> ()  [unwired: 2 in, 2 out]
            n322 = property on="Quit" class="Bool (strict)"("Disabled"=w279) -> ()  [unwired: 2 in, 2 out]
            n323 = property on="DeleteChannel" class="Bool (strict)"("Disabled"=w279) -> ()  [unwired: 2 in, 2 out]
            n324 = property on="WriteToFile" class="Bool (strict)"("Disabled"=w279) -> ()  [unwired: 2 in, 2 out]
            n325 = property on="CurrentModulationB" class="Bool (strict)"("Disabled"=w279) -> ()  [unwired: 2 in, 2 out]
            n326 = property on="SetCurrentB" class="Bool (strict)"("Disabled"=w279) -> ()  [unwired: 2 in, 2 out]
            n327 = property on="SetOutputOnB" class="Bool (strict)"("Disabled"=w279) -> ()  [unwired: 2 in, 2 out]
            n328 = property on="SetVoltageB" class="Bool (strict)"("Disabled"=w279) -> ()  [unwired: 2 in, 2 out]
            n329 = property on="SetOutputOffB" class="Bool (strict)"("Disabled"=w279) -> ()  [unwired: 2 in, 2 out]
            n330 = property on="SetVoltageAll" class="Bool (strict)"("Disabled"=w279) -> ()  [unwired: 2 in, 2 out]
            n331 = property on="SetCurrentAll" class="Bool (strict)"("Disabled"=w279) -> ()  [unwired: 2 in, 2 out]
            n332 = property on="DisconnectAll" class="Bool (strict)"("Disabled"=w279) -> ()  [unwired: 2 in, 2 out]
          }
        }
        n333 = Merge Errors(w257) -> (w255:errorcluster)
      }
      event "ConnectAll": Value Change {
        n334 = event-data() -> ()  [unwired: 7 out]
        n335 = flat-sequence {
          tunnel: [w285] -> w282
          tunnel: [w294] -> w283
          tunnel: w282 -> [w294]
          frame #0 {
            w284 = u8 2 ("Disabled")
            n336 = property on="Quit" class="Bool (strict)"("Disabled"=w284) -> ()  [unwired: 2 in, 2 out]
            n337 = property on="ReadFromFile" class="Bool (strict)"("Disabled"=w284) -> ()  [unwired: 2 in, 2 out]
            n338 = property on="CurrentModulationB" class="Bool (strict)"("Disabled"=w284) -> ()  [unwired: 2 in, 2 out]
            n339 = property on="WriteToFile" class="Bool (strict)"("Disabled"=w284) -> ()  [unwired: 2 in, 2 out]
            n340 = property on="ConnectAll" class="Bool (strict)"("Disabled"=w284) -> ()  [unwired: 2 in, 2 out]
            n341 = property on="Set Output ON All" class="Bool (strict)"("Disabled"=w284) -> ()  [unwired: 2 in, 2 out]
            n342 = property on="SetOutputOffB" class="Bool (strict)"("Disabled"=w284) -> ()  [unwired: 2 in, 2 out]
            n343 = property on="AddChannel" class="Bool (strict)"("Disabled"=w284) -> ()  [unwired: 2 in, 2 out]
            n344 = property on="DisconnectChannel" class="Bool (strict)"("Disabled"=w284) -> ()  [unwired: 2 in, 2 out]
            n345 = property on="SetCurrentAll" class="Bool (strict)"("Disabled"=w284) -> ()  [unwired: 2 in, 2 out]
            n346 = property on="SetOutputOnB" class="Bool (strict)"("Disabled"=w284) -> ()  [unwired: 2 in, 2 out]
            n347 = property on="ConnectChannel" class="Bool (strict)"("Disabled"=w284) -> ()  [unwired: 2 in, 2 out]
            n348 = property on="DeleteChannel" class="Bool (strict)"("Disabled"=w284) -> ()  [unwired: 2 in, 2 out]
            n349 = property on="SetCurrentB" class="Bool (strict)"("Disabled"=w284) -> ()  [unwired: 2 in, 2 out]
            n350 = property on="SetVoltageB" class="Bool (strict)"("Disabled"=w284) -> ()  [unwired: 2 in, 2 out]
            n351 = property on="SetVoltageAll" class="Bool (strict)"("Disabled"=w284) -> ()  [unwired: 2 in, 2 out]
            n352 = property on="DisconnectAll" class="Bool (strict)"("Disabled"=w284) -> ()  [unwired: 2 in, 2 out]
          }
          frame #1 {
            n353 = local read "VIRef"() -> (w287:refnum<vi>[])
            n354 = Array Size(array=w287) -> (size(s)=w286:i32)
            n355 = for {
              N: w286 -> [_]
              tunnel: [w288] -> w285 mode=indexing
              i -> [w289]
              n356 = local read "VIRef"() -> (w292:refnum<vi>[])
              n357 = Index Array(array=w292, index=w289) -> (element=w291:refnum<vi>)
              n358 = invoke class="VI" method="Ctrl Val.Set"(reference=w291, "Control Name"="Connect", "Value"=TRUE ("OK Button")) -> (error out=w288:errorcluster)  [unwired: 2 in, 4 out]
            }
          }
          frame #2 {
            w295 = u8 0 ("Disabled")
            n359 = local write "ConnectAll"(FALSE ("ConnectChannel")) -> ()
            n360 = property on="Quit" class="Bool (strict)"("Disabled"=w295) -> ()  [unwired: 2 in, 2 out]
            n361 = property on="AddChannel" class="Bool (strict)"("Disabled"=w295) -> ()  [unwired: 2 in, 2 out]
            n362 = property on="DisconnectChannel" class="Bool (strict)"("Disabled"=w295) -> ()  [unwired: 2 in, 2 out]
            n363 = property on="ConnectAll" class="Bool (strict)"("Disabled"=w295) -> ()  [unwired: 2 in, 2 out]
            n364 = property on="Set Output ON All" class="Bool (strict)"("Disabled"=w295) -> ()  [unwired: 2 in, 2 out]
            n365 = property on="SetOutputOffB" class="Bool (strict)"("Disabled"=w295) -> ()  [unwired: 2 in, 2 out]
            n366 = property on="SetCurrentAll" class="Bool (strict)"("Disabled"=w295) -> ()  [unwired: 2 in, 2 out]
            n367 = property on="ConnectChannel" class="Bool (strict)"("Disabled"=w295) -> ()  [unwired: 2 in, 2 out]
            n368 = property on="SetVoltageAll" class="Bool (strict)"("Disabled"=w295) -> ()  [unwired: 2 in, 2 out]
            n369 = property on="SetOutputOnB" class="Bool (strict)"("Disabled"=w295) -> ()  [unwired: 2 in, 2 out]
            n370 = property on="CurrentModulationB" class="Bool (strict)"("Disabled"=w295) -> ()  [unwired: 2 in, 2 out]
            n371 = property on="DisconnectAll" class="Bool (strict)"("Disabled"=w295) -> ()  [unwired: 2 in, 2 out]
            n372 = property on="ReadFromFile" class="Bool (strict)"("Disabled"=w295) -> ()  [unwired: 2 in, 2 out]
            n373 = property on="WriteToFile" class="Bool (strict)"("Disabled"=w295) -> ()  [unwired: 2 in, 2 out]
            n374 = property on="SetCurrentB" class="Bool (strict)"("Disabled"=w295) -> ()  [unwired: 2 in, 2 out]
            n375 = property on="SetVoltageB" class="Bool (strict)"("Disabled"=w295) -> ()  [unwired: 2 in, 2 out]
            n376 = property on="DeleteChannel" class="Bool (strict)"("Disabled"=w295) -> ()  [unwired: 2 in, 2 out]
          }
        }
        n377 = Merge Errors(w283) -> (w281:errorcluster)
      }
      event "DisconnectAll": Value Change {
        n378 = event-data() -> ()  [unwired: 7 out]
        n379 = flat-sequence {
          tunnel: [w301] -> w299
          tunnel: [w310] -> w298
          tunnel: w299 -> [w310]
          frame #0 {
            w300 = u8 2 ("Disabled")
            n380 = property on="Quit" class="Bool (strict)"("Disabled"=w300) -> ()  [unwired: 2 in, 2 out]
            n381 = property on="ReadFromFile" class="Bool (strict)"("Disabled"=w300) -> ()  [unwired: 2 in, 2 out]
            n382 = property on="CurrentModulationB" class="Bool (strict)"("Disabled"=w300) -> ()  [unwired: 2 in, 2 out]
            n383 = property on="ConnectAll" class="Bool (strict)"("Disabled"=w300) -> ()  [unwired: 2 in, 2 out]
            n384 = property on="ConnectChannel" class="Bool (strict)"("Disabled"=w300) -> ()  [unwired: 2 in, 2 out]
            n385 = property on="AddChannel" class="Bool (strict)"("Disabled"=w300) -> ()  [unwired: 2 in, 2 out]
            n386 = property on="DisconnectChannel" class="Bool (strict)"("Disabled"=w300) -> ()  [unwired: 2 in, 2 out]
            n387 = property on="Set Output ON All" class="Bool (strict)"("Disabled"=w300) -> ()  [unwired: 2 in, 2 out]
            n388 = property on="WriteToFile" class="Bool (strict)"("Disabled"=w300) -> ()  [unwired: 2 in, 2 out]
            n389 = property on="SetOutputOffB" class="Bool (strict)"("Disabled"=w300) -> ()  [unwired: 2 in, 2 out]
            n390 = property on="SetCurrentAll" class="Bool (strict)"("Disabled"=w300) -> ()  [unwired: 2 in, 2 out]
            n391 = property on="SetOutputOnB" class="Bool (strict)"("Disabled"=w300) -> ()  [unwired: 2 in, 2 out]
            n392 = property on="DeleteChannel" class="Bool (strict)"("Disabled"=w300) -> ()  [unwired: 2 in, 2 out]
            n393 = property on="SetCurrentB" class="Bool (strict)"("Disabled"=w300) -> ()  [unwired: 2 in, 2 out]
            n394 = property on="SetVoltageB" class="Bool (strict)"("Disabled"=w300) -> ()  [unwired: 2 in, 2 out]
            n395 = property on="SetVoltageAll" class="Bool (strict)"("Disabled"=w300) -> ()  [unwired: 2 in, 2 out]
            n396 = property on="DisconnectAll" class="Bool (strict)"("Disabled"=w300) -> ()  [unwired: 2 in, 2 out]
          }
          frame #1 {
            n397 = local read "VIRef"() -> (w303:refnum<vi>[])
            n398 = Array Size(array=w303) -> (size(s)=w302:i32)
            n399 = for {
              N: w302 -> [_]
              tunnel: [w304] -> w301 mode=indexing
              i -> [w305]
              n400 = local read "VIRef"() -> (w308:refnum<vi>[])
              n401 = Index Array(array=w308, index=w305) -> (element=w307:refnum<vi>)
              n402 = invoke class="VI" method="Ctrl Val.Set"(reference=w307, "Control Name"="Connect", "Value"=FALSE ("OK Button")) -> (error out=w304:errorcluster)  [unwired: 2 in, 4 out]
            }
          }
          frame #2 {
            w311 = u8 0 ("Disabled")
            n403 = local write "DisconnectAll"(FALSE ("ConnectChannel")) -> ()
            n404 = property on="Quit" class="Bool (strict)"("Disabled"=w311) -> ()  [unwired: 2 in, 2 out]
            n405 = property on="ConnectAll" class="Bool (strict)"("Disabled"=w311) -> ()  [unwired: 2 in, 2 out]
            n406 = property on="ConnectChannel" class="Bool (strict)"("Disabled"=w311) -> ()  [unwired: 2 in, 2 out]
            n407 = property on="AddChannel" class="Bool (strict)"("Disabled"=w311) -> ()  [unwired: 2 in, 2 out]
            n408 = property on="DisconnectChannel" class="Bool (strict)"("Disabled"=w311) -> ()  [unwired: 2 in, 2 out]
            n409 = property on="ReadFromFile" class="Bool (strict)"("Disabled"=w311) -> ()  [unwired: 2 in, 2 out]
            n410 = property on="Set Output ON All" class="Bool (strict)"("Disabled"=w311) -> ()  [unwired: 2 in, 2 out]
            n411 = property on="WriteToFile" class="Bool (strict)"("Disabled"=w311) -> ()  [unwired: 2 in, 2 out]
            n412 = property on="SetOutputOnB" class="Bool (strict)"("Disabled"=w311) -> ()  [unwired: 2 in, 2 out]
            n413 = property on="CurrentModulationB" class="Bool (strict)"("Disabled"=w311) -> ()  [unwired: 2 in, 2 out]
            n414 = property on="SetCurrentB" class="Bool (strict)"("Disabled"=w311) -> ()  [unwired: 2 in, 2 out]
            n415 = property on="SetVoltageB" class="Bool (strict)"("Disabled"=w311) -> ()  [unwired: 2 in, 2 out]
            n416 = property on="SetVoltageAll" class="Bool (strict)"("Disabled"=w311) -> ()  [unwired: 2 in, 2 out]
            n417 = property on="DisconnectAll" class="Bool (strict)"("Disabled"=w311) -> ()  [unwired: 2 in, 2 out]
            n418 = property on="DeleteChannel" class="Bool (strict)"("Disabled"=w311) -> ()  [unwired: 2 in, 2 out]
            n419 = property on="SetOutputOffB" class="Bool (strict)"("Disabled"=w311) -> ()  [unwired: 2 in, 2 out]
            n420 = property on="SetCurrentAll" class="Bool (strict)"("Disabled"=w311) -> ()  [unwired: 2 in, 2 out]
          }
        }
        n421 = Merge Errors(w298) -> (w297:errorcluster)
      }
      event "SetVoltageB": Value Change {
        n422 = event-data() -> ()  [unwired: 7 out]
        n423 = local write "SetVoltageB"(FALSE ("ConnectChannel")) -> ()
        n424 = flat-sequence {
          tunnel: [w319] -> w315
          tunnel: [w328] -> w314
          tunnel: w315 -> [w328]
          frame #0 {
            w317 = u8 2 ("Disabled")
            n425 = property on="Quit" class="Bool (strict)"("Disabled"=w317) -> ()  [unwired: 2 in, 2 out]
            n426 = property on="AddChannel" class="Bool (strict)"("Disabled"=w317) -> ()  [unwired: 2 in, 2 out]
            n427 = property on="Set Output ON All" class="Bool (strict)"("Disabled"=w317) -> ()  [unwired: 2 in, 2 out]
            n428 = property on="CurrentModulationB" class="Bool (strict)"("Disabled"=w317) -> ()  [unwired: 2 in, 2 out]
            n429 = property on="ConnectAll" class="Bool (strict)"("Disabled"=w317) -> ()  [unwired: 2 in, 2 out]
            n430 = property on="DisconnectChannel" class="Bool (strict)"("Disabled"=w317) -> ()  [unwired: 2 in, 2 out]
            n431 = property on="ReadFromFile" class="Bool (strict)"("Disabled"=w317) -> ()  [unwired: 2 in, 2 out]
            n432 = property on="ConnectChannel" class="Bool (strict)"("Disabled"=w317) -> ()  [unwired: 2 in, 2 out]
            n433 = property on="DeleteChannel" class="Bool (strict)"("Disabled"=w317) -> ()  [unwired: 2 in, 2 out]
            n434 = property on="WriteToFile" class="Bool (strict)"("Disabled"=w317) -> ()  [unwired: 2 in, 2 out]
            n435 = property on="SetCurrentB" class="Bool (strict)"("Disabled"=w317) -> ()  [unwired: 2 in, 2 out]
            n436 = property on="SetOutputOnB" class="Bool (strict)"("Disabled"=w317) -> ()  [unwired: 2 in, 2 out]
            n437 = property on="SetVoltageB" class="Bool (strict)"("Disabled"=w317) -> ()  [unwired: 2 in, 2 out]
            n438 = property on="SetOutputOffB" class="Bool (strict)"("Disabled"=w317) -> ()  [unwired: 2 in, 2 out]
            n439 = property on="SetVoltageAll" class="Bool (strict)"("Disabled"=w317) -> ()  [unwired: 2 in, 2 out]
            n440 = property on="SetCurrentAll" class="Bool (strict)"("Disabled"=w317) -> ()  [unwired: 2 in, 2 out]
            n441 = property on="DisconnectAll" class="Bool (strict)"("Disabled"=w317) -> ()  [unwired: 2 in, 2 out]
          }
          frame #1 {
            n442 = property on="List of channels" class="MCListbox (strict)"() -> ("Value"=w318:i32)  [unwired: 2 in, 2 out]
            n443 = local read "VIRef"() -> (w326:refnum<vi>[])
            n444 = local read "SetVoltage"() -> (w324:dbl)
            n445 = Index Array(array=w326, index=w318) -> (element=w325:refnum<vi>)
            n446 = invoke class="VI" method="Ctrl Val.Set"(reference=w325, "Control Name"="SetVoltage", "Value"=w324) -> (reference out=w321:refnum<vi>, error out=w320:errorcluster)  [unwired: 2 in, 3 out]
            n447 = invoke class="VI" method="Ctrl Val.Set"(reference=w321, error in=w320, "Control Name"="NeedToSetVoltage", "Value"=TRUE ("ConnectChannel")) -> (error out=w319:errorcluster)  [unwired: 1 in, 4 out]
          }
          frame #2 {
            w329 = u8 0 ("Disabled")
            n448 = property on="Quit" class="Bool (strict)"("Disabled"=w329) -> ()  [unwired: 2 in, 2 out]
            n449 = property on="ConnectAll" class="Bool (strict)"("Disabled"=w329) -> ()  [unwired: 2 in, 2 out]
            n450 = property on="Set Output ON All" class="Bool (strict)"("Disabled"=w329) -> ()  [unwired: 2 in, 2 out]
            n451 = property on="AddChannel" class="Bool (strict)"("Disabled"=w329) -> ()  [unwired: 2 in, 2 out]
            n452 = property on="CurrentModulationB" class="Bool (strict)"("Disabled"=w329) -> ()  [unwired: 2 in, 2 out]
            n453 = property on="DisconnectChannel" class="Bool (strict)"("Disabled"=w329) -> ()  [unwired: 2 in, 2 out]
            n454 = property on="ReadFromFile" class="Bool (strict)"("Disabled"=w329) -> ()  [unwired: 2 in, 2 out]
            n455 = property on="ConnectChannel" class="Bool (strict)"("Disabled"=w329) -> ()  [unwired: 2 in, 2 out]
            n456 = property on="DeleteChannel" class="Bool (strict)"("Disabled"=w329) -> ()  [unwired: 2 in, 2 out]
            n457 = property on="SetVoltageAll" class="Bool (strict)"("Disabled"=w329) -> ()  [unwired: 2 in, 2 out]
            n458 = property on="SetCurrentAll" class="Bool (strict)"("Disabled"=w329) -> ()  [unwired: 2 in, 2 out]
            n459 = property on="DisconnectAll" class="Bool (strict)"("Disabled"=w329) -> ()  [unwired: 2 in, 2 out]
            n460 = property on="WriteToFile" class="Bool (strict)"("Disabled"=w329) -> ()  [unwired: 2 in, 2 out]
            n461 = property on="SetCurrentB" class="Bool (strict)"("Disabled"=w329) -> ()  [unwired: 2 in, 2 out]
            n462 = property on="SetOutputOnB" class="Bool (strict)"("Disabled"=w329) -> ()  [unwired: 2 in, 2 out]
            n463 = property on="SetVoltageB" class="Bool (strict)"("Disabled"=w329) -> ()  [unwired: 2 in, 2 out]
            n464 = property on="SetOutputOffB" class="Bool (strict)"("Disabled"=w329) -> ()  [unwired: 2 in, 2 out]
          }
        }
        n465 = Merge Errors(w314) -> (w313:errorcluster)
      }
      event "SetOutputOnB": Value Change {
        n466 = event-data() -> ()  [unwired: 2 out]
        n467 = property on="List of channels" class="MCListbox (strict)"() -> ("Value"=w333:i32)  [unwired: 2 in, 2 out]
        n468 = flat-sequence {
          tunnel: w333 -> [w335]
          tunnel: [w335] -> w332
          tunnel: w332 -> [w342]
          tunnel: [w337] -> w331
          tunnel: [w347] -> w330
          tunnel: w331 -> [w347]
          frame #0 {
            w334 = u8 2 ("Disabled")
            n469 = property on="ConnectAll" class="Bool (strict)"("Disabled"=w334) -> ()  [unwired: 2 in, 2 out]
            n470 = property on="Set Output ON All" class="Bool (strict)"("Disabled"=w334) -> ()  [unwired: 2 in, 2 out]
            n471 = property on="AddChannel" class="Bool (strict)"("Disabled"=w334) -> ()  [unwired: 2 in, 2 out]
            n472 = property on="CurrentModulationB" class="Bool (strict)"("Disabled"=w334) -> ()  [unwired: 2 in, 2 out]
            n473 = property on="DisconnectChannel" class="Bool (strict)"("Disabled"=w334) -> ()  [unwired: 2 in, 2 out]
            n474 = property on="ReadFromFile" class="Bool (strict)"("Disabled"=w334) -> ()  [unwired: 2 in, 2 out]
            n475 = property on="Quit" class="Bool (strict)"("Disabled"=w334) -> ()  [unwired: 2 in, 2 out]
            n476 = property on="ConnectChannel" class="Bool (strict)"("Disabled"=w334) -> ()  [unwired: 2 in, 2 out]
            n477 = property on="DeleteChannel" class="Bool (strict)"("Disabled"=w334) -> ()  [unwired: 2 in, 2 out]
            n478 = property on="WriteToFile" class="Bool (strict)"("Disabled"=w334) -> ()  [unwired: 2 in, 2 out]
            n479 = property on="SetCurrentB" class="Bool (strict)"("Disabled"=w334) -> ()  [unwired: 2 in, 2 out]
            n480 = property on="SetOutputOnB" class="Bool (strict)"("Disabled"=w334) -> ()  [unwired: 2 in, 2 out]
            n481 = property on="SetVoltageB" class="Bool (strict)"("Disabled"=w334) -> ()  [unwired: 2 in, 2 out]
            n482 = property on="SetOutputOffB" class="Bool (strict)"("Disabled"=w334) -> ()  [unwired: 2 in, 2 out]
            n483 = property on="SetVoltageAll" class="Bool (strict)"("Disabled"=w334) -> ()  [unwired: 2 in, 2 out]
            n484 = property on="SetCurrentAll" class="Bool (strict)"("Disabled"=w334) -> ()  [unwired: 2 in, 2 out]
            n485 = property on="DisconnectAll" class="Bool (strict)"("Disabled"=w334) -> ()  [unwired: 2 in, 2 out]
          }
          frame #1 {
            n486 = local read "VIRef"() -> (w345:refnum<vi>[])
            n487 = local write "SetOutputOnB"(FALSE ("ConnectChannel")) -> ()
            n488 = Index Array(array=w345, index=w342) -> (element=w344:refnum<vi>)
            n489 = invoke class="VI" method="Ctrl Val.Set"(reference=w344, "Control Name"="SetOutput", "Value"=TRUE ("ConnectChannel")) -> (reference out=w339:refnum<vi>, error out=w338:errorcluster)  [unwired: 2 in, 3 out]
            n490 = invoke class="VI" method="Ctrl Val.Set"(reference=w339, error in=w338, "Control Name"="NeedToSetOutput", "Value"=TRUE ("ConnectChannel")) -> (error out=w337:errorcluster)  [unwired: 1 in, 4 out]
          }
          frame #2 {
            w348 = u8 0 ("Disabled")
            n491 = property on="ConnectAll" class="Bool (strict)"("Disabled"=w348) -> ()  [unwired: 2 in, 2 out]
            n492 = property on="Set Output ON All" class="Bool (strict)"("Disabled"=w348) -> ()  [unwired: 2 in, 2 out]
            n493 = property on="AddChannel" class="Bool (strict)"("Disabled"=w348) -> ()  [unwired: 2 in, 2 out]
            n494 = property on="DisconnectChannel" class="Bool (strict)"("Disabled"=w348) -> ()  [unwired: 2 in, 2 out]
            n495 = property on="ReadFromFile" class="Bool (strict)"("Disabled"=w348) -> ()  [unwired: 2 in, 2 out]
            n496 = property on="ConnectChannel" class="Bool (strict)"("Disabled"=w348) -> ()  [unwired: 2 in, 2 out]
            n497 = property on="Quit" class="Bool (strict)"("Disabled"=w348) -> ()  [unwired: 2 in, 2 out]
            n498 = property on="DeleteChannel" class="Bool (strict)"("Disabled"=w348) -> ()  [unwired: 2 in, 2 out]
            n499 = property on="SetOutputOffB" class="Bool (strict)"("Disabled"=w348) -> ()  [unwired: 2 in, 2 out]
            n500 = property on="CurrentModulationB" class="Bool (strict)"("Disabled"=w348) -> ()  [unwired: 2 in, 2 out]
            n501 = property on="SetVoltageAll" class="Bool (strict)"("Disabled"=w348) -> ()  [unwired: 2 in, 2 out]
            n502 = property on="SetCurrentAll" class="Bool (strict)"("Disabled"=w348) -> ()  [unwired: 2 in, 2 out]
            n503 = property on="DisconnectAll" class="Bool (strict)"("Disabled"=w348) -> ()  [unwired: 2 in, 2 out]
            n504 = property on="WriteToFile" class="Bool (strict)"("Disabled"=w348) -> ()  [unwired: 2 in, 2 out]
            n505 = property on="SetCurrentB" class="Bool (strict)"("Disabled"=w348) -> ()  [unwired: 2 in, 2 out]
            n506 = property on="SetOutputOnB" class="Bool (strict)"("Disabled"=w348) -> ()  [unwired: 2 in, 2 out]
            n507 = property on="SetVoltageB" class="Bool (strict)"("Disabled"=w348) -> ()  [unwired: 2 in, 2 out]
          }
        }
      }
      event "Set Output ON All": Value Change {
        n508 = event-data() -> ("NewVal"=w349:bool)  [unwired: 1 out]
        n509 = flat-sequence {
          tunnel: [w354] -> w350
          tunnel: w349 -> [w354]
          tunnel: [w359] -> w352
          tunnel: w350 -> [w356]
          tunnel: [w370] -> w353
          tunnel: w352 -> [w370]
          frame #0 {
            w355 = u8 2 ("Disabled")
            n510 = property on="Quit" class="Bool (strict)"("Disabled"=w355) -> ()  [unwired: 2 in, 2 out]
            n511 = property on="AddChannel" class="Bool (strict)"("Disabled"=w355) -> ()  [unwired: 2 in, 2 out]
            n512 = property on="CurrentModulationB" class="Bool (strict)"("Disabled"=w355) -> ()  [unwired: 2 in, 2 out]
            n513 = property on="DisconnectChannel" class="Bool (strict)"("Disabled"=w355) -> ()  [unwired: 2 in, 2 out]
            n514 = property on="ConnectAll" class="Bool (strict)"("Disabled"=w355) -> ()  [unwired: 2 in, 2 out]
            n515 = property on="ReadFromFile" class="Bool (strict)"("Disabled"=w355) -> ()  [unwired: 2 in, 2 out]
            n516 = property on="ConnectChannel" class="Bool (strict)"("Disabled"=w355) -> ()  [unwired: 2 in, 2 out]
            n517 = property on="DeleteChannel" class="Bool (strict)"("Disabled"=w355) -> ()  [unwired: 2 in, 2 out]
            n518 = property on="WriteToFile" class="Bool (strict)"("Disabled"=w355) -> ()  [unwired: 2 in, 2 out]
            n519 = property on="SetCurrentB" class="Bool (strict)"("Disabled"=w355) -> ()  [unwired: 2 in, 2 out]
            n520 = property on="SetOutputOnB" class="Bool (strict)"("Disabled"=w355) -> ()  [unwired: 2 in, 2 out]
            n521 = property on="SetVoltageB" class="Bool (strict)"("Disabled"=w355) -> ()  [unwired: 2 in, 2 out]
            n522 = property on="SetOutputOffB" class="Bool (strict)"("Disabled"=w355) -> ()  [unwired: 2 in, 2 out]
            n523 = property on="SetVoltageAll" class="Bool (strict)"("Disabled"=w355) -> ()  [unwired: 2 in, 2 out]
            n524 = property on="SetCurrentAll" class="Bool (strict)"("Disabled"=w355) -> ()  [unwired: 2 in, 2 out]
            n525 = property on="DisconnectAll" class="Bool (strict)"("Disabled"=w355) -> ()  [unwired: 2 in, 2 out]
          }
          frame #1 {
            n526 = local read "VIRef"() -> (w358:refnum<vi>[])
            n527 = Array Size(array=w358) -> (size(s)=w357:i32)
            n528 = for {
              N: w357 -> [_]
              tunnel: [w361] -> w359 mode=indexing
              tunnel: w356 -> [w360]
              i -> [w363]
              n529 = local read "VIRef"() -> (w368:refnum<vi>[])
              n530 = Index Array(array=w368, index=w363) -> (element=w367:refnum<vi>)
              n531 = invoke class="VI" method="Ctrl Val.Set"(reference=w367, "Control Name"="SetOutput", "Value"=w360) -> (reference out=w364:refnum<vi>, error out=w362:errorcluster)  [unwired: 2 in, 3 out]
              n532 = invoke class="VI" method="Ctrl Val.Set"(reference=w364, error in=w362, "Control Name"="NeedToSetOutput", "Value"=TRUE ("ConnectChannel")) -> (error out=w361:errorcluster)  [unwired: 1 in, 4 out]
            }
          }
          frame #2 {
            w371 = u8 0 ("Disabled")
            n533 = disable-structure shown="Disabled" {
              frame Disabled {
                n534 = local write "Set Output ON All"(FALSE ("ConnectChannel")) -> ()
              }
              frame Enabled {
              }
            }
            n535 = property on="Quit" class="Bool (strict)"("Disabled"=w371) -> ()  [unwired: 2 in, 2 out]
            n536 = property on="ConnectAll" class="Bool (strict)"("Disabled"=w371) -> ()  [unwired: 2 in, 2 out]
            n537 = property on="Set Output ON All" class="Bool (strict)"("Disabled"=w371) -> ()  [unwired: 2 in, 2 out]
            n538 = property on="AddChannel" class="Bool (strict)"("Disabled"=w371) -> ()  [unwired: 2 in, 2 out]
            n539 = property on="DisconnectChannel" class="Bool (strict)"("Disabled"=w371) -> ()  [unwired: 2 in, 2 out]
            n540 = property on="ReadFromFile" class="Bool (strict)"("Disabled"=w371) -> ()  [unwired: 2 in, 2 out]
            n541 = property on="ConnectChannel" class="Bool (strict)"("Disabled"=w371) -> ()  [unwired: 2 in, 2 out]
            n542 = property on="DeleteChannel" class="Bool (strict)"("Disabled"=w371) -> ()  [unwired: 2 in, 2 out]
            n543 = property on="SetVoltageB" class="Bool (strict)"("Disabled"=w371) -> ()  [unwired: 2 in, 2 out]
            n544 = property on="CurrentModulationB" class="Bool (strict)"("Disabled"=w371) -> ()  [unwired: 2 in, 2 out]
            n545 = property on="SetOutputOffB" class="Bool (strict)"("Disabled"=w371) -> ()  [unwired: 2 in, 2 out]
            n546 = property on="SetVoltageAll" class="Bool (strict)"("Disabled"=w371) -> ()  [unwired: 2 in, 2 out]
            n547 = property on="SetCurrentAll" class="Bool (strict)"("Disabled"=w371) -> ()  [unwired: 2 in, 2 out]
            n548 = property on="DisconnectAll" class="Bool (strict)"("Disabled"=w371) -> ()  [unwired: 2 in, 2 out]
            n549 = property on="WriteToFile" class="Bool (strict)"("Disabled"=w371) -> ()  [unwired: 2 in, 2 out]
            n550 = property on="SetCurrentB" class="Bool (strict)"("Disabled"=w371) -> ()  [unwired: 2 in, 2 out]
            n551 = property on="SetOutputOnB" class="Bool (strict)"("Disabled"=w371) -> ()  [unwired: 2 in, 2 out]
          }
        }
        n552 = Merge Errors(w353) -> (w351:errorcluster)
      }
      event "SetOutputOffB": Value Change {
        n553 = event-data() -> ()  [unwired: 7 out]
        n554 = local write "SetOutputOffB"(FALSE ("ConnectChannel")) -> ()
        n555 = property on="List of channels" class="MCListbox (strict)"() -> ("Value"=w377:i32)  [unwired: 2 in, 2 out]
        n556 = flat-sequence {
          tunnel: w377 -> [w379]
          tunnel: [w379] -> w376
          tunnel: w376 -> [w386]
          tunnel: [w380] -> w373
          tunnel: [w390] -> w374
          tunnel: w373 -> [w390]
          frame #0 {
            w378 = u8 2 ("Disabled")
            n557 = property on="ConnectAll" class="Bool (strict)"("Disabled"=w378) -> ()  [unwired: 2 in, 2 out]
            n558 = property on="Set Output ON All" class="Bool (strict)"("Disabled"=w378) -> ()  [unwired: 2 in, 2 out]
            n559 = property on="AddChannel" class="Bool (strict)"("Disabled"=w378) -> ()  [unwired: 2 in, 2 out]
            n560 = property on="CurrentModulationB" class="Bool (strict)"("Disabled"=w378) -> ()  [unwired: 2 in, 2 out]
            n561 = property on="DisconnectChannel" class="Bool (strict)"("Disabled"=w378) -> ()  [unwired: 2 in, 2 out]
            n562 = property on="ReadFromFile" class="Bool (strict)"("Disabled"=w378) -> ()  [unwired: 2 in, 2 out]
            n563 = property on="Quit" class="Bool (strict)"("Disabled"=w378) -> ()  [unwired: 2 in, 2 out]
            n564 = property on="ConnectChannel" class="Bool (strict)"("Disabled"=w378) -> ()  [unwired: 2 in, 2 out]
            n565 = property on="DeleteChannel" class="Bool (strict)"("Disabled"=w378) -> ()  [unwired: 2 in, 2 out]
            n566 = property on="WriteToFile" class="Bool (strict)"("Disabled"=w378) -> ()  [unwired: 2 in, 2 out]
            n567 = property on="SetCurrentB" class="Bool (strict)"("Disabled"=w378) -> ()  [unwired: 2 in, 2 out]
            n568 = property on="SetOutputOnB" class="Bool (strict)"("Disabled"=w378) -> ()  [unwired: 2 in, 2 out]
            n569 = property on="SetVoltageB" class="Bool (strict)"("Disabled"=w378) -> ()  [unwired: 2 in, 2 out]
            n570 = property on="SetOutputOffB" class="Bool (strict)"("Disabled"=w378) -> ()  [unwired: 2 in, 2 out]
            n571 = property on="SetVoltageAll" class="Bool (strict)"("Disabled"=w378) -> ()  [unwired: 2 in, 2 out]
            n572 = property on="SetCurrentAll" class="Bool (strict)"("Disabled"=w378) -> ()  [unwired: 2 in, 2 out]
            n573 = property on="DisconnectAll" class="Bool (strict)"("Disabled"=w378) -> ()  [unwired: 2 in, 2 out]
          }
          frame #1 {
            n574 = local read "VIRef"() -> (w388:refnum<vi>[])
            n575 = Index Array(array=w388, index=w386) -> (element=w387:refnum<vi>)
            n576 = invoke class="VI" method="Ctrl Val.Set"(reference=w387, "Control Name"="SetOutput", "Value"=FALSE ("ConnectChannel")) -> (reference out=w383:refnum<vi>, error out=w381:errorcluster)  [unwired: 2 in, 3 out]
            n577 = invoke class="VI" method="Ctrl Val.Set"(reference=w383, error in=w381, "Control Name"="NeedToSetOutput", "Value"=TRUE ("ConnectChannel")) -> (error out=w380:errorcluster)  [unwired: 1 in, 4 out]
          }
          frame #2 {
            w391 = u8 0 ("Disabled")
            n578 = property on="ConnectAll" class="Bool (strict)"("Disabled"=w391) -> ()  [unwired: 2 in, 2 out]
            n579 = property on="Set Output ON All" class="Bool (strict)"("Disabled"=w391) -> ()  [unwired: 2 in, 2 out]
            n580 = property on="AddChannel" class="Bool (strict)"("Disabled"=w391) -> ()  [unwired: 2 in, 2 out]
            n581 = property on="CurrentModulationB" class="Bool (strict)"("Disabled"=w391) -> ()  [unwired: 2 in, 2 out]
            n582 = property on="DisconnectChannel" class="Bool (strict)"("Disabled"=w391) -> ()  [unwired: 2 in, 2 out]
            n583 = property on="ReadFromFile" class="Bool (strict)"("Disabled"=w391) -> ()  [unwired: 2 in, 2 out]
            n584 = property on="ConnectChannel" class="Bool (strict)"("Disabled"=w391) -> ()  [unwired: 2 in, 2 out]
            n585 = property on="Quit" class="Bool (strict)"("Disabled"=w391) -> ()  [unwired: 2 in, 2 out]
            n586 = property on="DeleteChannel" class="Bool (strict)"("Disabled"=w391) -> ()  [unwired: 2 in, 2 out]
            n587 = property on="SetOutputOffB" class="Bool (strict)"("Disabled"=w391) -> ()  [unwired: 2 in, 2 out]
            n588 = property on="SetVoltageAll" class="Bool (strict)"("Disabled"=w391) -> ()  [unwired: 2 in, 2 out]
            n589 = property on="SetCurrentAll" class="Bool (strict)"("Disabled"=w391) -> ()  [unwired: 2 in, 2 out]
            n590 = property on="DisconnectAll" class="Bool (strict)"("Disabled"=w391) -> ()  [unwired: 2 in, 2 out]
            n591 = property on="WriteToFile" class="Bool (strict)"("Disabled"=w391) -> ()  [unwired: 2 in, 2 out]
            n592 = property on="SetCurrentB" class="Bool (strict)"("Disabled"=w391) -> ()  [unwired: 2 in, 2 out]
            n593 = property on="SetOutputOnB" class="Bool (strict)"("Disabled"=w391) -> ()  [unwired: 2 in, 2 out]
            n594 = property on="SetVoltageB" class="Bool (strict)"("Disabled"=w391) -> ()  [unwired: 2 in, 2 out]
          }
        }
      }
      event "WriteToFile": Value Change {
        n595 = event-data() -> ()  [unwired: 7 out]
        n596 = local read "ADRESS"() -> (w396:string[])
        n597 = Array Size(array=w396) -> (size(s)=w395:i32)
        n598 = flat-sequence {
          tunnel: w395 -> [w405]
          tunnel: [w397] -> w393
          tunnel: [w438] -> w394
          tunnel: w393 -> [w438]
          frame #0 {
            n599 = Number To Decimal String(number=w405) -> (decimal integer string=w400:string)  [unwired: 1 out]
            n600 = Write to Text File(text=w400) -> (refnum out=w399:refnum<file>, cancelled=w398:bool, error out=w401:errorcluster)  [unwired: 1 in, 2 out]
            n601 = Write to Text File(file (use dialog)=w399, text="\nИМЯ  АДРЕС  ТОК  НАПРЯЖЕНИЕ", error in=w401) -> (refnum out=w402:refnum<file>, error out=w403:errorcluster)  [unwired: 2 out]
            n602 = for {
              N: w405 -> [_]
              tunnel: w398 -> [w415]
              tunnel: w403 -> [w410]
              tunnel: w402 -> [w417]
              tunnel: [w408] -> w397 mode=indexing
              i -> [w416]
              w421 = "" ("Control Name")
              w427 = "\t"
              n603 = local read "VIRef"() -> (w425:refnum<vi>[])
              n604 = Index Array(array=w425, index=w416) -> (element=w424:refnum<vi>)
              n605 = invoke class="VI" method="Ctrl Val.Get"(reference=w424, "Control Name"="SetVoltageStr") -> (reference out=w419:refnum<vi>, error out=w412:errorcluster, "Get Control Value Variant"=w426:variant)  [unwired: 2 in, 1 out]
              n606 = invoke class="VI" method="Ctrl Val.Get"(reference=w419, error in=w412, "Control Name"="SetCurrentStr") -> (error out=w411:errorcluster, "Get Control Value Variant"=w422:variant)  [unwired: 1 in, 2 out]
              n607 = local read "ADRESS"() -> (w432:string[])
              n608 = local read "NAME"() -> (w430:string[])
              n609 = Index Array(array=w430, index=w416) -> (element=w428:string)
              n610 = Index Array(array=w432, index=w416) -> (element=w431:string)
              n611 = Variant To Data(type=w421, Variant=w422) -> (data=w407:string, error out=w414:errorcluster)  [unwired: 1 in]
              n612 = Variant To Data(type=w421, Variant=w426) -> (data=w406:string, error out=w413:errorcluster)  [unwired: 1 in]
              n613 = Merge Errors(w411, w414, w413, w410) -> (w409:errorcluster)
              n614 = Concatenate Strings("\r\n", w428, w427, w431, w427, w407, w427, w406) -> (w418:string)
              n615 = case shown="True" w415 {
                tunnel: w417 -> [w435 _]
                tunnel: w418 -> [w436 _]
                tunnel: w409 -> [w434 w437]
                tunnel: [w433 w437] -> w408
                frame False {
                  n616 = Write to Text File(file (use dialog)=w435, text=w436, error in=w434) -> (error out=w433:errorcluster)  [unwired: 3 out]
                }
                frame True {
                }
              }
            }
          }
          frame #1 {
            n617 = local write "WriteToFile"(FALSE ("ConnectChannel")) -> ()
          }
        }
        n618 = Merge Errors(w394) -> (w392:errorcluster)
      }
      event "ReadFromFile": Value Change {
        n619 = event-data() -> ()  [unwired: 2 out]
        n620 = local read "ReadFromFile"() -> (w442:bool)
        n621 = Read from Text File(count=100) -> (text=w446:string[], cancelled=w445:bool, error out=w444:errorcluster)  [unwired: 1 in, 3 out]
        n622 = Not(x=w445) -> (.not. x?=w441:bool)
        n623 = And(x=w442, y=w441) -> (x .and. y?=w440:bool)
        n624 = case shown="True" w440 {
          tunnel: w446 -> [_ w450]
          tunnel: w444 -> [w448 w452]
          tunnel: [w448 w451] -> w443
          frame False {
            n625 = local write "ReadFromFile"(FALSE ("ConnectChannel")) -> ()
          }
          frame True {
            n626 = flat-sequence {
              tunnel: w452 -> [w460]
              tunnel: [w459] -> w454
              tunnel: w454 -> [w469]
              tunnel: [w469] -> w453
              tunnel: w453 -> [_]
              tunnel: [w480] -> w456
              tunnel: w450 -> [w479]
              tunnel: w456 -> [w514]
              tunnel: [w514] -> w455
              frame #0 {
                w458 = u8 2 ("Disabled")
                n627 = local read "VIRef"() -> (w461:refnum<vi>[])
                n628 = property on="Set Output ON All" class="Bool (strict)"("Disabled"=w458) -> ()  [unwired: 2 in, 2 out]
                n629 = property on="CurrentModulationB" class="Bool (strict)"("Disabled"=w458) -> ()  [unwired: 2 in, 2 out]
                n630 = property on="ConnectAll" class="Bool (strict)"("Disabled"=w458) -> ()  [unwired: 2 in, 2 out]
                n631 = property on="ReadFromFile" class="Bool (strict)"("Disabled"=w458) -> ()  [unwired: 2 in, 2 out]
                n632 = property on="ConnectChannel" class="Bool (strict)"("Disabled"=w458) -> ()  [unwired: 2 in, 2 out]
                n633 = property on="DisconnectChannel" class="Bool (strict)"("Disabled"=w458) -> ()  [unwired: 2 in, 2 out]
                n634 = property on="WriteToFile" class="Bool (strict)"("Disabled"=w458) -> ()  [unwired: 2 in, 2 out]
                n635 = property on="AddChannel" class="Bool (strict)"("Disabled"=w458) -> ()  [unwired: 2 in, 2 out]
                n636 = property on="SetOutputOnB" class="Bool (strict)"("Disabled"=w458) -> ()  [unwired: 2 in, 2 out]
                n637 = property on="Quit" class="Bool (strict)"("Disabled"=w458) -> ()  [unwired: 2 in, 2 out]
                n638 = property on="DeleteChannel" class="Bool (strict)"("Disabled"=w458) -> ()  [unwired: 2 in, 2 out]
                n639 = property on="SetCurrentB" class="Bool (strict)"("Disabled"=w458) -> ()  [unwired: 2 in, 2 out]
                n640 = property on="SetOutputOffB" class="Bool (strict)"("Disabled"=w458) -> ()  [unwired: 2 in, 2 out]
                n641 = property on="SetCurrentAll" class="Bool (strict)"("Disabled"=w458) -> ()  [unwired: 2 in, 2 out]
                n642 = property on="SetVoltageB" class="Bool (strict)"("Disabled"=w458) -> ()  [unwired: 2 in, 2 out]
                n643 = property on="SetVoltageAll" class="Bool (strict)"("Disabled"=w458) -> ()  [unwired: 2 in, 2 out]
                n644 = property on="DisconnectAll" class="Bool (strict)"("Disabled"=w458) -> ()  [unwired: 2 in, 2 out]
                n645 = Array Size(array=w461) -> (size(s)=w457:i32)
                n646 = for {
                  N: w457 -> [_]
                  tunnel: w461 -> [w465]
                  tunnel: w460 -> [w463]
                  tunnel: [w462] -> w459 mode=indexing
                  i -> [w466]
                  n647 = Index Array(array=w465, index=w466) -> (element=w464:refnum<vi>)
                  n648 = invoke class="VI" method="Ctrl Val.Set"(reference=w464, error in=w463, "Control Name"="Connect", "Value"=FALSE) -> (error out=w462:errorcluster)  [unwired: 1 in, 4 out]
                }
              }
              frame #1 {
                n649 = Wait (ms)(milliseconds to wait=u32 1000) -> ()  [unwired: 1 out]
              }
              frame #2 {
                n650 = local read "VIRef"() -> (w472:refnum<vi>[])
                n651 = Array Size(array=w472) -> (size(s)=w471:i32)
                n652 = for {
                  N: w471 -> [_]
                  tunnel: w472 -> [w474]
                  i -> [w475]
                  n653 = Index Array(array=w474, index=w475) -> (element=w473:refnum<vi>)
                  n654 = invoke class="VI" method="Abort VI"(reference=w473) -> ()  [unwired: 2 in, 3 out]
                }
              }
              frame #3 {
                w477 = string[] [] ("GlobalInAdress")
                n655 = Wait (ms)(milliseconds to wait=u32 250) -> ()  [unwired: 1 out]
                n656 = local write "NAME"(w477) -> ()
                n657 = local write "ADRESS"(w477) -> ()
                n658 = local write "VIRef"(refnum<vi>[] []) -> ()
              }
              frame #4 {
                n659 = Index Array(array=w479, index=0) -> (element=w483:string)
                n660 = Decimal String To Number(string=w483) -> (number=w481:i32)  [unwired: 3 out]
                n661 = for {
                  N: w481 -> [_]
                  tunnel: w479 -> [w508]
                  tunnel: [w484] -> w480 mode=indexing
                  i -> [w511]
                  n662 = Add(x=2, y=w511) -> (x+y=w510:i32)
                  n663 = Index Array(array=w508, index=w510) -> (element=w507:string)
                  n664 = Spreadsheet String To Array(format string="%s", spreadsheet string=w507, array type (2D Dbl)=string[] [] ("GlobalInAdress")) -> (array=w498:string[])  [unwired: 1 out]
                  n665 = Index Array(array=w498, index=3) -> (element=w496:string)
                  n666 = Index Array(array=w498, index=0) -> (element=w502:string)
                  n667 = Index Array(array=w498, index=1) -> (element=w503:string)
                  n668 = Index Array(array=w498, index=2) -> (element=w497:string)
                  n669 = local read "ADRESS"() -> (w494:string[])
                  n670 = Scan From String(input string=w496, default 1=0.0 ("default value 1")) -> (output 1=w489:dbl)  [unwired: 3 in, 3 out]
                  n671 = Scan From String(input string=w497, default 1=0.0 ("default value 1")) -> (output 1=w491:dbl)  [unwired: 3 in, 3 out]
                  n672 = local read "NAME"() -> (w495:string[])
                  n673 = local read "VIRef"() -> (w493:refnum<vi>[])
                  n674 = call "AddChannel.vi"("VIRef"=w493, "Name"=w502, "SetCurrent"=w489, "ADRESS"=w494, "NAME"=w495, "Address"=w503, "SetVoltage"=w491) -> ("NAMEOut"=w488:string[], "error out"=w485:errorcluster, "ADRESSOut"=w486:string[], "VIRefOut"=w487:refnum<vi>[])  [unwired: 1 in, 4 out]
                  n675 = local write "NAME"(w488) -> ()
                  n676 = local write "VIRef"(w487) -> ()
                  n677 = flat-sequence {
                    tunnel: w485 -> [w513]
                    tunnel: [w513] -> w484
                    frame #0 {
                      n678 = Wait (ms)(milliseconds to wait=u32 50) -> ()  [unwired: 1 out]
                    }
                  }
                  n679 = local write "ADRESS"(w486) -> ()
                }
              }
              frame #5 {
                w515 = u8 0 ("Disabled")
                n680 = local write "ReadFromFile"(FALSE ("ConnectChannel")) -> ()
                n681 = property on="ConnectAll" class="Bool (strict)"("Disabled"=w515) -> ()  [unwired: 2 in, 2 out]
                n682 = property on="Set Output ON All" class="Bool (strict)"("Disabled"=w515) -> ()  [unwired: 2 in, 2 out]
                n683 = property on="AddChannel" class="Bool (strict)"("Disabled"=w515) -> ()  [unwired: 2 in, 2 out]
                n684 = property on="CurrentModulationB" class="Bool (strict)"("Disabled"=w515) -> ()  [unwired: 2 in, 2 out]
                n685 = property on="DisconnectChannel" class="Bool (strict)"("Disabled"=w515) -> ()  [unwired: 2 in, 2 out]
                n686 = property on="ReadFromFile" class="Bool (strict)"("Disabled"=w515) -> ()  [unwired: 2 in, 2 out]
                n687 = property on="ConnectChannel" class="Bool (strict)"("Disabled"=w515) -> ()  [unwired: 2 in, 2 out]
                n688 = property on="DeleteChannel" class="Bool (strict)"("Disabled"=w515) -> ()  [unwired: 2 in, 2 out]
                n689 = property on="WriteToFile" class="Bool (strict)"("Disabled"=w515) -> ()  [unwired: 2 in, 2 out]
                n690 = property on="SetCurrentB" class="Bool (strict)"("Disabled"=w515) -> ()  [unwired: 2 in, 2 out]
                n691 = property on="Quit" class="Bool (strict)"("Disabled"=w515) -> ()  [unwired: 2 in, 2 out]
                n692 = property on="SetOutputOnB" class="Bool (strict)"("Disabled"=w515) -> ()  [unwired: 2 in, 2 out]
                n693 = property on="SetVoltageB" class="Bool (strict)"("Disabled"=w515) -> ()  [unwired: 2 in, 2 out]
                n694 = property on="SetOutputOffB" class="Bool (strict)"("Disabled"=w515) -> ()  [unwired: 2 in, 2 out]
                n695 = property on="SetVoltageAll" class="Bool (strict)"("Disabled"=w515) -> ()  [unwired: 2 in, 2 out]
                n696 = property on="SetCurrentAll" class="Bool (strict)"("Disabled"=w515) -> ()  [unwired: 2 in, 2 out]
                n697 = property on="DisconnectAll" class="Bool (strict)"("Disabled"=w515) -> ()  [unwired: 2 in, 2 out]
              }
            }
            n698 = Merge Errors(w455) -> (w451:errorcluster)
          }
        }
      }
      event "SetCurrentB": Value Change {
        n699 = event-data() -> ()  [unwired: 7 out]
        n700 = local write "SetCurrentB"(FALSE ("ConnectChannel")) -> ()
        n701 = property on="List of channels" class="MCListbox (strict)"() -> (error out=w519:errorcluster, "Value"=w523:i32)  [unwired: 2 in, 1 out]
        n702 = flat-sequence {
          tunnel: w523 -> [w526]
          tunnel: [w526] -> w522
          tunnel: [w524] -> w520
          tunnel: w519 -> [w524]
          tunnel: w522 -> [w528]
          tunnel: w520 -> [w527]
          tunnel: [w529] -> w518
          tunnel: [w538] -> w517
          tunnel: w518 -> [w538]
          frame #0 {
            w525 = u8 2 ("Disabled")
            n703 = property on="AddChannel" class="Bool (strict)"("Disabled"=w525) -> ()  [unwired: 2 in, 2 out]
            n704 = property on="Set Output ON All" class="Bool (strict)"("Disabled"=w525) -> ()  [unwired: 2 in, 2 out]
            n705 = property on="CurrentModulationB" class="Bool (strict)"("Disabled"=w525) -> ()  [unwired: 2 in, 2 out]
            n706 = property on="ConnectAll" class="Bool (strict)"("Disabled"=w525) -> ()  [unwired: 2 in, 2 out]
            n707 = property on="DisconnectChannel" class="Bool (strict)"("Disabled"=w525) -> ()  [unwired: 2 in, 2 out]
            n708 = property on="ReadFromFile" class="Bool (strict)"("Disabled"=w525) -> ()  [unwired: 2 in, 2 out]
            n709 = property on="Quit" class="Bool (strict)"("Disabled"=w525) -> ()  [unwired: 2 in, 2 out]
            n710 = property on="ConnectChannel" class="Bool (strict)"("Disabled"=w525) -> ()  [unwired: 2 in, 2 out]
            n711 = property on="DeleteChannel" class="Bool (strict)"("Disabled"=w525) -> ()  [unwired: 2 in, 2 out]
            n712 = property on="WriteToFile" class="Bool (strict)"("Disabled"=w525) -> ()  [unwired: 2 in, 2 out]
            n713 = property on="SetCurrentB" class="Bool (strict)"("Disabled"=w525) -> ()  [unwired: 2 in, 2 out]
            n714 = property on="SetOutputOnB" class="Bool (strict)"("Disabled"=w525) -> ()  [unwired: 2 in, 2 out]
            n715 = property on="SetVoltageB" class="Bool (strict)"("Disabled"=w525) -> ()  [unwired: 2 in, 2 out]
            n716 = property on="SetOutputOffB" class="Bool (strict)"("Disabled"=w525) -> ()  [unwired: 2 in, 2 out]
            n717 = property on="SetVoltageAll" class="Bool (strict)"("Disabled"=w525) -> ()  [unwired: 2 in, 2 out]
            n718 = property on="SetCurrentAll" class="Bool (strict)"("Disabled"=w525) -> ()  [unwired: 2 in, 2 out]
            n719 = property on="DisconnectAll" class="Bool (strict)"("Disabled"=w525) -> ()  [unwired: 2 in, 2 out]
          }
          frame #1 {
            n720 = local read "VIRef"() -> (w536:refnum<vi>[])
            n721 = local read "SetCurrent"() -> (w534:dbl)
            n722 = Index Array(array=w536, index=w528) -> (element=w535:refnum<vi>)
            n723 = invoke class="VI" method="Ctrl Val.Set"(reference=w535, error in=w527, "Control Name"="SetCurrent", "Value"=w534) -> (reference out=w531:refnum<vi>, error out=w530:errorcluster)  [unwired: 1 in, 3 out]
            n724 = invoke class="VI" method="Ctrl Val.Set"(reference=w531, error in=w530, "Control Name"="NeedToSetCurrent", "Value"=TRUE ("ConnectChannel")) -> (error out=w529:errorcluster)  [unwired: 1 in, 4 out]
          }
          frame #2 {
            w539 = u8 0 ("Disabled")
            n725 = property on="AddChannel" class="Bool (strict)"("Disabled"=w539) -> ()  [unwired: 2 in, 2 out]
            n726 = property on="Set Output ON All" class="Bool (strict)"("Disabled"=w539) -> ()  [unwired: 2 in, 2 out]
            n727 = property on="DisconnectChannel" class="Bool (strict)"("Disabled"=w539) -> ()  [unwired: 2 in, 2 out]
            n728 = property on="ConnectAll" class="Bool (strict)"("Disabled"=w539) -> ()  [unwired: 2 in, 2 out]
            n729 = property on="ReadFromFile" class="Bool (strict)"("Disabled"=w539) -> ()  [unwired: 2 in, 2 out]
            n730 = property on="ConnectChannel" class="Bool (strict)"("Disabled"=w539) -> ()  [unwired: 2 in, 2 out]
            n731 = property on="DeleteChannel" class="Bool (strict)"("Disabled"=w539) -> ()  [unwired: 2 in, 2 out]
            n732 = property on="Quit" class="Bool (strict)"("Disabled"=w539) -> ()  [unwired: 2 in, 2 out]
            n733 = property on="WriteToFile" class="Bool (strict)"("Disabled"=w539) -> ()  [unwired: 2 in, 2 out]
            n734 = property on="CurrentModulationB" class="Bool (strict)"("Disabled"=w539) -> ()  [unwired: 2 in, 2 out]
            n735 = property on="SetCurrentB" class="Bool (strict)"("Disabled"=w539) -> ()  [unwired: 2 in, 2 out]
            n736 = property on="SetOutputOnB" class="Bool (strict)"("Disabled"=w539) -> ()  [unwired: 2 in, 2 out]
            n737 = property on="SetVoltageB" class="Bool (strict)"("Disabled"=w539) -> ()  [unwired: 2 in, 2 out]
            n738 = property on="SetOutputOffB" class="Bool (strict)"("Disabled"=w539) -> ()  [unwired: 2 in, 2 out]
            n739 = property on="SetVoltageAll" class="Bool (strict)"("Disabled"=w539) -> ()  [unwired: 2 in, 2 out]
            n740 = property on="SetCurrentAll" class="Bool (strict)"("Disabled"=w539) -> ()  [unwired: 2 in, 2 out]
            n741 = property on="DisconnectAll" class="Bool (strict)"("Disabled"=w539) -> ()  [unwired: 2 in, 2 out]
          }
        }
      }
      event "DeleteChannel": Value Change {
        n742 = event-data() -> ()  [unwired: 7 out]
        n743 = property on="List of channels" class="MCListbox (strict)"() -> ("Value"=w543:i32)  [unwired: 2 in, 2 out]
        n744 = flat-sequence {
          tunnel: [w552] -> w544
          tunnel: w543 -> [w552]
          tunnel: [w556] -> w551
          tunnel: [w554] -> w550
          tunnel: [w555] -> w549
          tunnel: w544 -> [w554]
          tunnel: [w562] -> w548
          tunnel: w551 -> [w562]
          tunnel: [w561] -> w547
          tunnel: w550 -> [w561]
          tunnel: w549 -> [w560]
          tunnel: [w560] -> w546
          tunnel: w548 -> [w567]
          tunnel: [w566] -> w545
          tunnel: w547 -> [w566]
          tunnel: w546 -> [w565]
          tunnel: [w564] -> w541
          tunnel: w545 -> [w569]
          tunnel: [w568] -> w542
          tunnel: w541 -> [w568]
          tunnel: w542 -> [w577]
          tunnel: [w577] -> w540
          frame #0 {
            w553 = u8 2 ("Disabled")
            n745 = property on="AddChannel" class="Bool (strict)"("Disabled"=w553) -> ()  [unwired: 2 in, 2 out]
            n746 = property on="Set Output ON All" class="Bool (strict)"("Disabled"=w553) -> ()  [unwired: 2 in, 2 out]
            n747 = property on="CurrentModulationB" class="Bool (strict)"("Disabled"=w553) -> ()  [unwired: 2 in, 2 out]
            n748 = property on="ConnectAll" class="Bool (strict)"("Disabled"=w553) -> ()  [unwired: 2 in, 2 out]
            n749 = property on="DisconnectChannel" class="Bool (strict)"("Disabled"=w553) -> ()  [unwired: 2 in, 2 out]
            n750 = property on="ReadFromFile" class="Bool (strict)"("Disabled"=w553) -> ()  [unwired: 2 in, 2 out]
            n751 = property on="Quit" class="Bool (strict)"("Disabled"=w553) -> ()  [unwired: 2 in, 2 out]
            n752 = property on="ConnectChannel" class="Bool (strict)"("Disabled"=w553) -> ()  [unwired: 2 in, 2 out]
            n753 = property on="DeleteChannel" class="Bool (strict)"("Disabled"=w553) -> ()  [unwired: 2 in, 2 out]
            n754 = property on="WriteToFile" class="Bool (strict)"("Disabled"=w553) -> ()  [unwired: 2 in, 2 out]
            n755 = property on="SetCurrentB" class="Bool (strict)"("Disabled"=w553) -> ()  [unwired: 2 in, 2 out]
            n756 = property on="SetOutputOnB" class="Bool (strict)"("Disabled"=w553) -> ()  [unwired: 2 in, 2 out]
            n757 = property on="SetVoltageB" class="Bool (strict)"("Disabled"=w553) -> ()  [unwired: 2 in, 2 out]
            n758 = property on="SetOutputOffB" class="Bool (strict)"("Disabled"=w553) -> ()  [unwired: 2 in, 2 out]
            n759 = property on="SetVoltageAll" class="Bool (strict)"("Disabled"=w553) -> ()  [unwired: 2 in, 2 out]
            n760 = property on="SetCurrentAll" class="Bool (strict)"("Disabled"=w553) -> ()  [unwired: 2 in, 2 out]
            n761 = property on="DisconnectAll" class="Bool (strict)"("Disabled"=w553) -> ()  [unwired: 2 in, 2 out]
          }
          frame #1 {
            n762 = local read "VIRef"() -> (w558:refnum<vi>[])
            n763 = Index Array(array=w558, index=w554) -> (element=w556:refnum<vi>)
            n764 = invoke class="VI" method="Ctrl Val.Set"(reference=w556, "Control Name"="Connect", "Value"=FALSE ("OK Button")) -> (error out=w555:errorcluster)  [unwired: 2 in, 4 out]
          }
          frame #2 {
            n765 = Wait (ms)(milliseconds to wait=u32 1000) -> ()  [unwired: 1 out]
          }
          frame #3 {
            n766 = invoke class="VI" method="Abort VI"(reference=w567, error in=w565) -> (error out=w564:errorcluster)  [unwired: 1 in, 2 out]
          }
          frame #4 {
            w570 = 1 ("length")
            n767 = local read "NAME"() -> (w571:string[])
            n768 = local read "VIRef"() -> (w576:refnum<vi>[])
            n769 = Delete From Array(array=w576, length=w570, index=w569) -> (array with subset deleted=w573:refnum<vi>[])  [unwired: 1 out]
            n770 = Delete From Array(array=w571, length=w570, index=w569) -> (array with subset deleted=w572:string[])  [unwired: 1 out]
            n771 = local read "ADRESS"() -> (w575:string[])
            n772 = local write "VIRef"(w573) -> ()
            n773 = local write "NAME"(w572) -> ()
            n774 = Delete From Array(array=w575, length=w570, index=w569) -> (array with subset deleted=w574:string[])  [unwired: 1 out]
            n775 = local write "ADRESS"(w574) -> ()
          }
          frame #5 {
            w578 = u8 0 ("Disabled")
            n776 = local write "DeleteChannel"(FALSE ("DeleteChannel")) -> ()
            n777 = property on="AddChannel" class="Bool (strict)"("Disabled"=w578) -> ()  [unwired: 2 in, 2 out]
            n778 = property on="CurrentModulationB" class="Bool (strict)"("Disabled"=w578) -> ()  [unwired: 2 in, 2 out]
            n779 = property on="DisconnectChannel" class="Bool (strict)"("Disabled"=w578) -> ()  [unwired: 2 in, 2 out]
            n780 = property on="ReadFromFile" class="Bool (strict)"("Disabled"=w578) -> ()  [unwired: 2 in, 2 out]
            n781 = property on="ConnectChannel" class="Bool (strict)"("Disabled"=w578) -> ()  [unwired: 2 in, 2 out]
            n782 = property on="Quit" class="Bool (strict)"("Disabled"=w578) -> ()  [unwired: 2 in, 2 out]
            n783 = property on="DeleteChannel" class="Bool (strict)"("Disabled"=w578) -> ()  [unwired: 2 in, 2 out]
            n784 = property on="WriteToFile" class="Bool (strict)"("Disabled"=w578) -> ()  [unwired: 2 in, 2 out]
            n785 = property on="Set Output ON All" class="Bool (strict)"("Disabled"=w578) -> ()  [unwired: 2 in, 2 out]
            n786 = property on="SetCurrentB" class="Bool (strict)"("Disabled"=w578) -> ()  [unwired: 2 in, 2 out]
            n787 = property on="ConnectAll" class="Bool (strict)"("Disabled"=w578) -> ()  [unwired: 2 in, 2 out]
            n788 = property on="SetOutputOnB" class="Bool (strict)"("Disabled"=w578) -> ()  [unwired: 2 in, 2 out]
            n789 = property on="SetVoltageB" class="Bool (strict)"("Disabled"=w578) -> ()  [unwired: 2 in, 2 out]
            n790 = property on="SetOutputOffB" class="Bool (strict)"("Disabled"=w578) -> ()  [unwired: 2 in, 2 out]
            n791 = property on="SetVoltageAll" class="Bool (strict)"("Disabled"=w578) -> ()  [unwired: 2 in, 2 out]
            n792 = property on="SetCurrentAll" class="Bool (strict)"("Disabled"=w578) -> ()  [unwired: 2 in, 2 out]
            n793 = property on="DisconnectAll" class="Bool (strict)"("Disabled"=w578) -> ()  [unwired: 2 in, 2 out]
          }
        }
      }
    }
    n794 = call <vilib>:"General Error Handler.vi"("type of dialog (OK msg:1)"=u8 0 ("Disabled"), "error in (no error)"=w36) -> ()  [unwired: 14 out]
  }
  n795 = while {
    stop <- FALSE stop-if-true
    n796 = property on="AddChannel" class="Bool (strict)"() -> ("Disabled"=w586:u8)  [unwired: 2 in, 2 out]
    n797 = local read "Quit"() -> (w584:bool)
    n798 = Not(x=w584) -> (.not. x?=w583:bool)
    n799 = Equal?(x=w586, y=u8 0) -> (x = y?=w582:bool)
    n800 = And(x=w583, y=w582) -> (x .and. y?=w581:bool)
    n801 = case shown="True" w581 {
      frame False {
      }
      frame True {
        w590 = string[] [] ("GlobalInAdress")
        n802 = local read "VIRef"() -> (w599:refnum<vi>[])
        n803 = Array Size(array=w599) -> (size(s)=w589:i32)
        n804 = for {
          N: w589 -> [_]
          tunnel: w599 -> [w668]
          shift-right: [w667] -> w588
          shift-left: w590 -> [w666]
          shift-right: [w664] -> w587
          shift-left: w590 -> [w665]
          shift-right: [w655] -> w596
          shift-left: w590 -> [w656]
          shift-right: [w644] -> w595
          shift-left: w590 -> [w651]
          shift-right: [w648] -> w593
          shift-left: w590 -> [w628]
          shift-right: [w642] -> w592
          shift-left: w590 -> [w643]
          i -> [w624]
          w641 = "" ("Control Name")
          n805 = Index Array(array=w668, index=w624) -> (element=w627:refnum<vi>)
          n806 = invoke class="VI" method="Ctrl Val.Get"(reference=w627, "Control Name"="SetVoltageStr") -> (error out=w636:errorcluster, "Get Control Value Variant"=w654:variant)  [unwired: 2 in, 2 out]
          n807 = invoke class="VI" method="Ctrl Val.Get"(reference=w627, "Control Name"="SetCurrentStr") -> (error out=w635:errorcluster, "Get Control Value Variant"=w653:variant)  [unwired: 2 in, 2 out]
          n808 = invoke class="VI" method="Ctrl Val.Get"(reference=w627, "Control Name"="Error") -> (error out=w622:errorcluster, "Get Control Value Variant"=w629:variant)  [unwired: 2 in, 2 out]
          n809 = invoke class="VI" method="Ctrl Val.Get"(reference=w627, "Control Name"="GetCurrent") -> (error out=w638:errorcluster, "Get Control Value Variant"=w661:variant)  [unwired: 2 in, 2 out]
          n810 = invoke class="VI" method="Ctrl Val.Get"(reference=w627, "Control Name"="GetVoltage") -> (error out=w637:errorcluster, "Get Control Value Variant"=w662:variant)  [unwired: 2 in, 2 out]
          n811 = invoke class="VI" method="Ctrl Val.Get"(reference=w627, "Control Name"="Output") -> (error out=w634:errorcluster, "Get Control Value Variant"=w645:variant)  [unwired: 2 in, 2 out]
          n812 = invoke class="VI" method="Ctrl Val.Get"(reference=w627, "Control Name"="Active") -> (error out=w633:errorcluster, "Get Control Value Variant"=w650:variant)  [unwired: 2 in, 2 out]
          n813 = Variant To Data(type=w641, Variant=w654) -> (data=w601:string)  [unwired: 1 in, 1 out]
          n814 = Variant To Data(type=w641, Variant=w653) -> (data=w606:string)  [unwired: 1 in, 1 out]
          n815 = Merge Errors(w622, w638, w637, w636) -> (w632:errorcluster)
          n816 = Merge Errors(w635, w634, w633) -> (w631:errorcluster)
          n817 = Variant To Data(type=w641, Variant=w661) -> (data=w658:string)  [unwired: 1 in, 1 out]
          n818 = Variant To Data(type=w641, Variant=w662) -> (data=w659:string)  [unwired: 1 in, 1 out]
          n819 = Variant To Data "Out"(type=w641, Variant=w645) -> (data=w630:string)  [unwired: 1 in, 1 out]
          n820 = String Length(string=w601) -> (length=w602:i32)
          n821 = String Length(string=w606) -> (length=w609:i32)
          n822 = Variant To Data(type=FALSE, Variant=w629) -> (data=w617:bool)  [unwired: 1 in, 1 out]
          n823 = disable-structure shown="Enabled" {
            disable-tunnel: [w679 w680] -> w618
            disable-tunnel: _ -> [w678 _]
            disable-tunnel: w617 -> [w677 w680]
            frame Disabled {
              n824 = Or(x=w677, y=w678) -> (x .or. y?=w679:bool)
            }
            frame Enabled {
            }
          }
          n825 = case shown="6, Default" w602 {
            tunnel: [4 ("milliseconds to wait") 5 ("milliseconds to wait")] -> w603
            tunnel: [0 ("milliseconds to wait") 0 ("milliseconds to wait")] -> w604
            frame 6, Default {
            }
            frame 7 {
            }
          }
          n826 = Variant To Data "Active"(type=FALSE, Variant=w650) -> (data=w616:bool)  [unwired: 1 in, 1 out]
          n827 = case shown="7" w609 {
            tunnel: [4 ("milliseconds to wait") 5 ("milliseconds to wait")] -> w608
            tunnel: [0 ("milliseconds to wait") 0 ("milliseconds to wait")] -> w607
            frame 6, Default {
            }
            frame 7 {
            }
          }
          n828 = Build Array (concatenate)(w665, w658) -> (w664:string[])
          n829 = Build Array (concatenate)(w666, w659) -> (w667:string[])
          n830 = case shown="True" w618 {
            tunnel: w627 -> [_ w731]
            tunnel: w624 -> [w713 w719]
            tunnel: [w712 w717] -> w619
            frame False {
              n831 = Bundle(w713, "milliseconds to wait"=8) -> (w714:cluster{i32, "milliseconds to wait":i32})  [unwired: 1 in]
              n832 = property on="error" class="MCListbox (strict)"("ActiveCell"=w714, "CellBG"=u32 16777225) -> (error out=w712:errorcluster)  [unwired: 2 in, 1 out]
            }
            frame True {
              w721 = "Connect" ("Control Name")
              n833 = invoke class="VI" method="Ctrl Val.Set"(reference=w731, "Control Name"=w721, "Value"=FALSE ("OK Button")) -> (reference out=w723:refnum<vi>, error out=w726:errorcluster)  [unwired: 2 in, 3 out]
              n834 = flat-sequence {
                tunnel: w726 -> [w736]
                tunnel: [w736] -> w724
                tunnel: w723 -> [w734]
                tunnel: [w734] -> w722
                tunnel: w721 -> [w733]
                tunnel: [w733] -> w720
                tunnel: w719 -> [w732]
                tunnel: [w732] -> w718
                frame #0 {
                  n835 = Wait (ms)(milliseconds to wait=u32 2000) -> ()  [unwired: 1 out]
                }
              }
              n836 = Bundle(w718, "milliseconds to wait"=8) -> (w728:cluster{i32, "milliseconds to wait":i32})  [unwired: 1 in]
              n837 = invoke class="VI" method="Ctrl Val.Set"(reference=w722, error in=w724, "Control Name"=w720, "Value"=TRUE ("OK Button")) -> (error out=w717:errorcluster)  [unwired: 1 in, 4 out]
              n838 = property on="error" class="MCListbox (strict)"("ActiveCell"=w728, "CellBG"=u32 16711680) -> ()  [unwired: 2 in, 2 out]
            }
          }
          n839 = case shown="\"0\"" w630 {
            tunnel: ["+" ("Control Name") "" ("Control Name") "-" ("Control Name")] -> w621
            tunnel: w624 -> [w681 w686 w691]
            frame "1" {
              n840 = Bundle(w681, "milliseconds to wait"=6) -> (w683:cluster{i32, "milliseconds to wait":i32})  [unwired: 1 in]
              n841 = property on="out" class="MCListbox (strict)"("ActiveCell"=w683, "CellBG"=u32 5895331) -> ()  [unwired: 2 in, 2 out]
            }
            frame Default {
              n842 = Bundle(w686, "milliseconds to wait"=6) -> (w688:cluster{i32, "milliseconds to wait":i32})  [unwired: 1 in]
              n843 = property on="out" class="MCListbox (strict)"("ActiveCell"=w688, "CellBG"=u32 16777225) -> ()  [unwired: 2 in, 2 out]
            }
            frame "0" {
              n844 = Bundle(w691, "milliseconds to wait"=6) -> (w693:cluster{i32, "milliseconds to wait":i32})  [unwired: 1 in]
              n845 = property on="out" class="MCListbox (strict)"("ActiveCell"=w693, "CellBG"=u32 13816530) -> ()  [unwired: 2 in, 2 out]
            }
          }
          n846 = String Subset(string=w601, offset (0)=w604, length (rest)=w603) -> (substring=w600:string)
          n847 = String Subset(string=w606, offset (0)=w607, length (rest)=w608) -> (substring=w605:string)
          n848 = case shown="False" w616 {
            tunnel: ["-" ("Control Name") "+" ("Control Name")] -> w649
            tunnel: w624 -> [w698 w707]
            tunnel: w621 -> [_ w706]
            tunnel: ["?" ("Control Name") w706] -> w620
            frame False {
              n849 = Bundle(w698, "milliseconds to wait"=7) -> (w704:cluster{i32, "milliseconds to wait":i32})  [unwired: 1 in]
              n850 = property on="active" class="MCListbox (strict)"("ActiveCell"=w704, "CellBG"=u32 14869218) -> (error out=w699:errorcluster)  [unwired: 2 in, 1 out]
              n851 = Bundle(w698, "milliseconds to wait"=6) -> (w697:cluster{i32, "milliseconds to wait":i32})  [unwired: 1 in]
              n852 = property on="out" class="MCListbox (strict)"(error in=w699, "ActiveCell"=w697, "CellBG"=u32 14869218) -> ()  [unwired: 1 in, 2 out]
            }
            frame True {
              n853 = Bundle(w707, "milliseconds to wait"=7) -> (w709:cluster{i32, "milliseconds to wait":i32})  [unwired: 1 in]
              n854 = property on="active" class="MCListbox (strict)"("ActiveCell"=w709, "CellBG"=u32 5895331) -> ()  [unwired: 2 in, 2 out]
            }
          }
          n855 = Merge Errors(w632, w631, w619) -> (w626:errorcluster)
          n856 = Search and Replace String(input string=w600, search string=",", replace string="." ("replace string (\"\")")) -> (result string=w613:string)  [unwired: 5 in, 3 out]
          n857 = Search and Replace String(input string=w605, search string=",", replace string="." ("replace string (\"\")")) -> (result string=w611:string)  [unwired: 5 in, 3 out]
          n858 = Build Array (concatenate)(w656, w613) -> (w655:string[])
          n859 = Build Array (concatenate)(w651, w611) -> (w644:string[])
          n860 = Build Array (concatenate)(w643, w620) -> (w642:string[])
          n861 = Build Array (concatenate)(w628, w649) -> (w648:string[])
          n862 = call <vilib>:"General Error Handler.vi"("type of dialog (OK msg:1)"=u32 0 ("milliseconds to wait"), "error in (no error)"=w626) -> ()  [unwired: 9 in, 5 out]
        }
        n863 = local read "ADRESS"() -> (w597:string[])
        n864 = local read "NAME"() -> (w594:string[])
        n865 = Build Array(w594, w597, w588, w587, w596, w595, w592, w593) -> (w598:string[][])
        n866 = Transpose 2D Array(2D array=w598) -> (transposed array=w591:string[][])
        n867 = property on="List of channels" class="MCListbox (strict)"("ItemNames"=w591) -> ()  [unwired: 2 in, 2 out]
      }
    }
  }
  n868 = property on="Set Output ON All" class="Bool (strict)"("Disabled"=w19) -> (error out=w11:errorcluster)  [unwired: 2 in, 1 out]
  n869 = property on="SetCurrentAll" class="Bool (strict)"("Disabled"=w19) -> ()  [unwired: 2 in, 2 out]
  n870 = property on="AddChannel" class="Bool (strict)"("Disabled"=w19) -> (error out=w18:errorcluster)  [unwired: 2 in, 1 out]
  n871 = property on="AddChannel" class="Bool (strict)"("Disabled"=u8 0) -> ()  [unwired: 2 in, 2 out]
  n872 = local write "текущий ист."(u8 0 ("текущий ист.")) -> ()
  n873 = property on="IP" class="Str"("Value"="" ("IP")) -> ()  [unwired: 2 in, 2 out]
  n874 = property on="№" class="Str"("Value"="" ("Name")) -> ()  [unwired: 2 in, 2 out]
  n875 = local write "WriteToFile"(w22) -> ()
  n876 = local write "DisconnectChannel"(w22) -> ()
  n877 = local write "ConnectChannel"(w22) -> ()
  n878 = local write "SetCurrentB"(w22) -> ()
  n879 = local write "ReadFromFile"(w22) -> ()
  n880 = local write "AddChannel"(w22) -> ()
  n881 = local write "Quit"(w22) -> ()
  n882 = local write "SetCurrentAll"(w22) -> ()
  n883 = local write "SetVoltageAll"(w22) -> ()
  n884 = local write "DeleteChannel"(w22) -> ()
  n885 = local write "SetVoltageB"(w22) -> ()
  n886 = local write "SetOutputOnB"(w21) -> ()
  n887 = local write "ConnectAll"(w21) -> ()
  n888 = local write "SetOutputOffB"(w21) -> ()
  n889 = local write "DisconnectAll"(w21) -> ()
  n890 = local write "CurrentModulationB"(w21) -> ()
  n891 = local write "CurrentModulationOn"(w21) -> ()
  n892 = for "инициализация цветов и размера ячеек табл." {
    N: 50 -> [_]
    i -> [w739]
    n893 = flat-sequence {
      tunnel: w739 -> [w744]
      tunnel: [w744] -> w738
      tunnel: w738 -> [w783]
      tunnel: [w783] -> w737
      tunnel: w737 -> [w796]
      frame #0 {
        w740 = "Application font" ("Font Name")
        n894 = Bundle(w744, 4) -> (w756:cluster{i32, i32})  [unwired: 1 in]
        n895 = property on="active" class="MCListbox (strict)"("ActiveCell"=w756, "Height"=u32 35 ("Active Cell:Cell Size:Height"), "CellFontSize"=u16 28 ("Size")) -> ()  [unwired: 2 in, 2 out]
        n896 = Bundle(w744, 6) -> (w742:cluster{i32, i32})  [unwired: 1 in]
        n897 = Bundle(w744, 5) -> (w741:cluster{i32, i32})  [unwired: 1 in]
        n898 = Bundle(w744, 0) -> (w767:cluster{i32, i32})  [unwired: 1 in]
        n899 = Bundle(w744, 2) -> (w743:cluster{i32, i32})  [unwired: 1 in]
        n900 = Bundle(w744, 3) -> (w757:cluster{i32, i32})  [unwired: 1 in]
        n901 = Bundle(w744, 1) -> (w766:cluster{i32, i32})  [unwired: 1 in]
        n902 = property on="active" class="MCListbox (strict)"("ActiveCell"=w742, "Height"=u32 35 ("Active Cell:Cell Size:Height"), "CellFontSize"=u16 28 ("Size"), "CellFontName"=w740) -> ()  [unwired: 2 in, 2 out]
        n903 = property on="active" class="MCListbox (strict)"("ActiveCell"=w741, "Height"=u32 35 ("Active Cell:Cell Size:Height"), "CellFontSize"=u16 28 ("Size"), "CellFontName"=w740) -> ()  [unwired: 2 in, 2 out]
        n904 = property on="active" class="MCListbox (strict)"("ActiveCell"=w767, "Height"=u32 35 ("Active Cell:Cell Size:Height"), "CellFontSize"=u16 28 ("Size"), "CellFontName"=w740) -> ()  [unwired: 2 in, 2 out]
        n905 = property on="active" class="MCListbox (strict)"("ActiveCell"=w743, "Height"=u32 35 ("Active Cell:Cell Size:Height"), "CellFontSize"=u16 28 ("Size"), "CellFontName"=w740) -> ()  [unwired: 2 in, 2 out]
        n906 = property on="active" class="MCListbox (strict)"("ActiveCell"=w757, "Height"=u32 35 ("Active Cell:Cell Size:Height"), "CellFontSize"=u16 28 ("Size"), "CellFontName"=w740) -> ()  [unwired: 2 in, 2 out]
        n907 = property on="active" class="MCListbox (strict)"("ActiveCell"=w766, "Height"=u32 35 ("Active Cell:Cell Size:Height"), "CellFontSize"=u16 28 ("Size"), "CellFontName"=w740) -> ()  [unwired: 2 in, 2 out]
      }
      frame #1 {
        w779 = T2 {"Font Name"="Application font", "Size"=28, "Bold"=FALSE, "Italic"=FALSE, "Underline"=FALSE, "Strikeout"=FALSE, "Color"=6908265} ("Active Cell:Cell Font")
        w774 = T2 {"Font Name"="Application font", "Size"=30, "Bold"=TRUE, "Italic"=FALSE, "Underline"=FALSE, "Strikeout"=FALSE, "Color"=2263842} ("Active Cell:Cell Font")
        n908 = Bundle(w783, 4) -> (w776:cluster{i32, i32})  [unwired: 1 in]
        n909 = Bundle(w783, 3) -> (w770:cluster{i32, i32})  [unwired: 1 in]
        n910 = Bundle(w783, 2) -> (w773:cluster{i32, i32})  [unwired: 1 in]
        n911 = Bundle(w783, 0) -> (w781:cluster{i32, i32})  [unwired: 1 in]
        n912 = Bundle(w783, 5) -> (w777:cluster{i32, i32})  [unwired: 1 in]
        n913 = property on="active" class="MCListbox (strict)"("ActiveCell"=w776, "CellFont"=w779) -> ()  [unwired: 2 in, 2 out]
        n914 = property on="active" class="MCListbox (strict)"("ActiveCell"=w770, "CellFont"=w774) -> ()  [unwired: 2 in, 2 out]
        n915 = property on="active" class="MCListbox (strict)"("ActiveCell"=w773, "CellFont"=w774) -> ()  [unwired: 2 in, 2 out]
        n916 = property on="active" class="MCListbox (strict)"("ActiveCell"=w781, "CellFont"=T2 {"Font Name"="Application font", "Size"=28, "Bold"=FALSE, "Italic"=FALSE, "Underline"=FALSE, "Strikeout"=FALSE, "Color"=0} ("Active Cell:Cell Font")) -> ()  [unwired: 2 in, 2 out]
        n917 = property on="active" class="MCListbox (strict)"("ActiveCell"=w777, "CellFont"=w779) -> ()  [unwired: 2 in, 2 out]
      }
      frame #2 {
        w795 = T2 {"Font Name"="Application font", "Size"=28, "Bold"=FALSE, "Italic"=FALSE, "Underline"=FALSE, "Strikeout"=FALSE, "Color"=0} ("Active Cell:Cell Font")
        n918 = Bundle(w796, 6) -> (w790:cluster{i32, i32})  [unwired: 1 in]
        n919 = Bundle(w796, 8) -> (w791:cluster{i32, i32})  [unwired: 1 in]
        n920 = Bundle(w796, 7) -> (w792:cluster{i32, i32})  [unwired: 1 in]
        n921 = property on="active" class="MCListbox (strict)"("ActiveCell"=w790, "CellBG"=u32 16777225) -> (error out=w789:errorcluster)  [unwired: 2 in, 1 out]
        n922 = property on="error" class="MCListbox (strict)"("ActiveCell"=w791, "CellBG"=u32 16777225) -> ()  [unwired: 2 in, 2 out]
        n923 = property on="out" class="MCListbox (strict)"("ActiveCell"=w792, "CellBG"=u32 16777225) -> (error out=w793:errorcluster)  [unwired: 2 in, 1 out]
        n924 = property on="active" class="MCListbox (strict)"(error in=w789, "ActiveCell"=w790, "CellFont"=w795) -> ()  [unwired: 1 in, 2 out]
        n925 = property on="active" class="MCListbox (strict)"(error in=w793, "ActiveCell"=w792, "CellFont"=w795) -> ()  [unwired: 1 in, 2 out]
      }
    }
  }
  n926 = property on="CurrentModulationB" class="Bool (strict)"(error in=w18, "Disabled"=w19) -> (error out=w17:errorcluster)  [unwired: 1 in, 1 out]
  n927 = property on="DisconnectAll" class="Bool (strict)"(error in=w11, "Disabled"=w19) -> (error out=w10:errorcluster)  [unwired: 1 in, 1 out]
  n928 = property on="DisconnectChannel" class="Bool (strict)"(error in=w17, "Disabled"=w19) -> (error out=w16:errorcluster)  [unwired: 1 in, 1 out]
  n929 = property on="WriteToFile" class="Bool (strict)"(error in=w10, "Disabled"=w19) -> (error out=w9:errorcluster)  [unwired: 1 in, 1 out]
  n930 = property on="SetCurrentB" class="Bool (strict)"(error in=w9, "Disabled"=w19) -> (error out=w8:errorcluster)  [unwired: 1 in, 1 out]
  n931 = property on="ConnectAll" class="Bool (strict)"(error in=w16, "Disabled"=w19) -> (error out=w15:errorcluster)  [unwired: 1 in, 1 out]
  n932 = property on="Quit" class="Bool (strict)"(error in=w8, "Disabled"=w19) -> (error out=w7:errorcluster)  [unwired: 1 in, 1 out]
  n933 = property on="ReadFromFile" class="Bool (strict)"(error in=w15, "Disabled"=w19) -> (error out=w14:errorcluster)  [unwired: 1 in, 1 out]
  n934 = property on="SetOutputOnB" class="Bool (strict)"(error in=w7, "Disabled"=w19) -> (error out=w6:errorcluster)  [unwired: 1 in, 1 out]
  n935 = property on="ConnectChannel" class="Bool (strict)"(error in=w14, "Disabled"=w19) -> (error out=w13:errorcluster)  [unwired: 1 in, 1 out]
  n936 = property on="SetVoltageB" class="Bool (strict)"(error in=w6, "Disabled"=w19) -> (error out=w5:errorcluster)  [unwired: 1 in, 1 out]
  n937 = property on="SetOutputOffB" class="Bool (strict)"(error in=w5, "Disabled"=w19) -> ()  [unwired: 1 in, 2 out]
  n938 = property on="DeleteChannel" class="Bool (strict)"(error in=w13, "Disabled"=w19) -> (error out=w12:errorcluster)  [unwired: 1 in, 1 out]
  n939 = property on="SetVoltageAll" class="Bool (strict)"(error in=w12, "Disabled"=w19) -> ()  [unwired: 1 in, 2 out]
  "VIRef" <- refnum<vi>[] []
  "ADRESS" <- string[] [] ("GlobalInAdress")
  "NAME" <- string[] [] ("GlobalInAdress")
  "CURRENTSET" <- dbl[] [] ("GlobalInAdress")
